vi "Periodic Tasks.vi"(8 "error in":errorcluster) -> ()   [LabVIEW 2019]
doc: "This VI runs in parallel to other tasks. It can contain as many user-defined periodic loops as you need. These can carry out PID or other sorts of timed response."
uses:
  <vilib>/Rock Robotics/WPI/Solenoid/WPI_SolenoidValue.ctl
  <vilib>/Rock Robotics/WPI/DriverStation/WPI_DriverStationRobotMode2.ctl
  Robot Global Data.vi
  <vilib>/Rock Robotics/WPI/ThirdParty/Phoenix-LabVIEW/Motor Controller/Sensor/CTRE_Phoenix_MotorControl_SetIntegratedSensorPosition_TalonFX.vi
  <vilib>/Rock Robotics/WPI/ThirdParty/Phoenix-LabVIEW/Motor Controller/Get/CTRE_Phoenix_MotorController_GetSelectedSensorData.vi
  <vilib>/Rock Robotics/WPI/Utilities/WPI_GetSetVariantRefNum.vi
  <vilib>/Rock Robotics/WPI/Solenoid/WPI_SolenoidSetEnum.vi
  <vilib>/Rock Robotics/WPI/ThirdParty/Phoenix-LabVIEW/Motor Controller/Get/CTRE_Phoenix_MotorController_GetQuadratureData.vi
  <vilib>/Rock Robotics/Network Tables/NT Read Numeric Array.vi
  <vilib>/Rock Robotics/Network Tables/NT Read String Array.vi
  <vilib>/Rock Robotics/Network Tables/NT Read Boolean Array.vi
  <vilib>/Rock Robotics/Network Tables/NT Write Numeric Array.vi
  <vilib>/Rock Robotics/Network Tables/NT Write String Array.vi
  <vilib>/Rock Robotics/Network Tables/NT Write Boolean Array.vi
  <vilib>/Rock Robotics/Network Tables/NT Read Number.vi
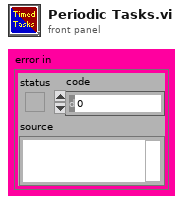
[diagram p1: front panel]
types:
  T1 = typedef "WPI_MotorControlDeviceRef.ctl" = cluster{"DeviceStatus":errorcluster, "Type":T2, "PWM":cluster{"PWM Channel":T3, "DeadBand":T4}, "CAN":cluster{"Device Number":u8, "SetOutput VI Ref":variant, "GetOutput VI Ref":variant, "Enable VI Ref":variant, "Disable VI Ref":variant, "Data":variant}, "Invert":bool, "DIO PWM":cluster{"PWM \"Enable\" Channel":T3, "DIOChannel":T5, "PWM Rate":dbl}}
  T2 = typedef "WPI_MotorControlType.ctl" = enum16{"PWM", "CAN", "DIO PWM"}
  T3 = typedef "FPGA_DIOPWMChannel.ctl" = enum8{"PWM 0", "PWM 1", "PWM 2", "PWM 3", "PWM 4", "PWM 5", "PWM 6", "PWM 7", "PWM 8", "PWM 9", "PWM MXP 0", "PWM MXP 1", "PWM MXP 2", "PWM MXP 3", "PWM MXP 4", "PWM MXP 5", "PWM MXP 6", "PWM MXP 7", "PWM MXP 8", "PWM MXP 9", "Invalid"}
  T4 = typedef "WPI_PWMDeadband.ctl" = cluster{"Name":string, "maxPositivePwm":i32, "minPositivePwm":i32, "centerPwm":i32, "maxNegativePwm":i32, "minNegativePwm":i32, "angularRange":u16}
  T5 = typedef "FPGA_DIOChannel.ctl" = enum8{"DIO 0", "DIO 1", "DIO 2", "DIO 3", "DIO 4", "DIO 5", "DIO 6", "DIO 7", "DIO 8", "DIO 9", "DIO MXP 0", "DIO MXP 1", "DIO MXP 2", "DIO MXP 3", "DIO MXP 4", "DIO MXP 5", "DIO MXP 6", "DIO MXP 7", "DIO MXP 8", "DIO MXP 9", "DIO MXP 10", "DIO MXP 11", "DIO MXP 12", "DIO MXP 13", "DIO MXP 14", "DIO MXP 15", "SPI Port CS1", "SPI Port CS2", "SPI Port CS3", "SPI Port MISO", "SPI Port MOSI", "Invalid"}
  T6 = typedef "WPI_DriverStationRobotMode2.ctl" = enum16{"Autonomous Disabled", "Autonomous Enabled", "Teleop Disabled", "Teleop Enabled", "Disconnected", "Finish", "Test Disabled", "Test Enabled", "Emergency Stopped"}
  T7 = typedef "WPI_AccelerometerDevRef.ctl" = cluster{"DevStatus":errorcluster, "Scaling":T8, "Analog Channels":T9, "I2C Bus":T11, "SPI Bus":T12, "Accel Range":T13, "ADXL Axes":T14, "Handle":i32, "Device Address":u8, "Accel Type":enum16{"Analog", "ADXL345 I2C", "ADXL345 SPI", "Internal", "ADXL362 SPI"}}
  T8 = typedef "WPI_AccelerometerScaling.ctl" = cluster{"Gain (VoltsPerG)":dbl, "Center Voltage":dbl}
  T9 = typedef "WPI_AccelerometerAnalogChannels.ctl" = cluster{"X-Axis":T10, "Y-Axis":T10, "Z-Axis":T10}
  T10 = typedef "FPGA_AIChannel.ctl" = enum8{"AI 0", "AI 1", "AI 2", "AI 3", "AI MXP 0", "AI MXP 1", "AI MXP 2", "AI MXP 3", "Invalid"}
  T11 = typedef "i2c_bus.ctl" = enum16{"I2C On-Board", "I2C MXP", "Invalid"}
  T12 = typedef "spi_bus.ctl" = enum16{"SPI On-Board, CS0", "SPI On-Board, CS1", "SPI On-Board, CS2", "SPI On-Board, CS3", "SPI MXP", "Invalid"}
  T13 = typedef "ADXL345 Range.ctl" = u8
  T14 = typedef "WPI_AccelerometerADXL345 Axes.ctl" = cluster{"X-Axis":bool, "Y-Axis":bool, "Z-Axis":bool}
  T15 = cluster{"X-Axis":dbl, "Y-Axis":dbl, "Z-Axis":dbl}
  T16 = typedef "WPI_SolenoidDevRef.ctl" = cluster{"DevStatus":errorcluster, "Pneumatics Control Module":u8, "Forward Solenoid Channel":T17, "Reverse Solenoid Channel":T17}
  T17 = typedef "WPI_SolenoidChannel.ctl" = enum8{"Solenoid 0", "Solenoid 1", "Solenoid 2", "Solenoid 3", "Solenoid 4", "Solenoid 5", "Solenoid 6", "Solenoid 7", "Invalid"}
  T18 = typedef "WPI_SolenoidValue.ctl" = enum16{"Off", "On", "Forward", "Reverse"}
  T19 = typedef "WPI_PotentiometerDevRef.ctl" = cluster{"DevStatus":errorcluster, "Analog Channel":T10, "Invert Output":bool}
  T20 = typedef "WPI_JoystickDevRef.ctl" = cluster{"Device":T21}
  T21 = typedef "WPI_JoystickDeviceEnum.ctl" = enum16{"USB 0", "USB 1", "USB 2", "USB 3", "USB 4", "USB 5"}
  T22 = typedef "Color Sensor V3 DevRef.ctl" = cluster{"I2CDevRef":T23}
  T23 = typedef "WPI_I2CDevRef.ctl" = cluster{"DevStatus":errorcluster, "Device Address":u8, "Handle":i32, "I2C Bus":T11}
  T24 = typedef "WPI_RobotDriveDevRef.ctl" = cluster{"DevStatus":errorcluster, "Motors[]":T1[], "Square Inputs":bool, "Max Output":dbl}
  T25 = cluster{"JoystickDevRef":T20, "RobotDriveDevRef":T24}
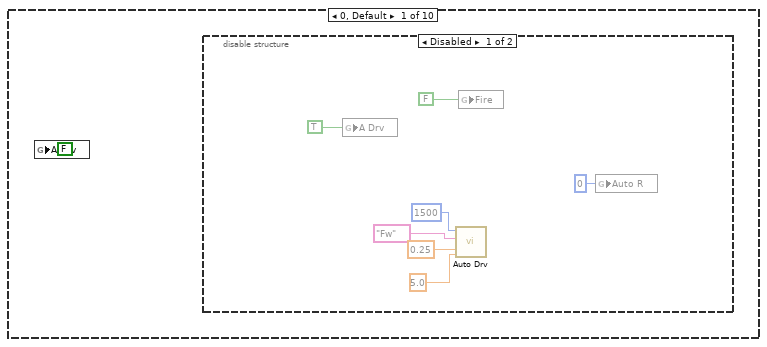
[diagram p2: hidden frame]
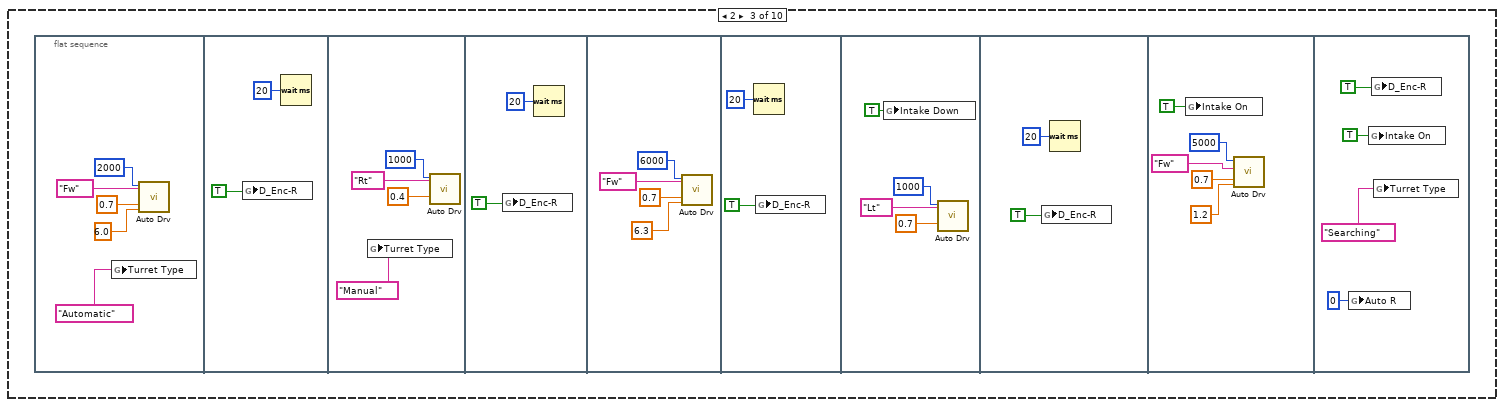
[diagram p4: hidden frame]
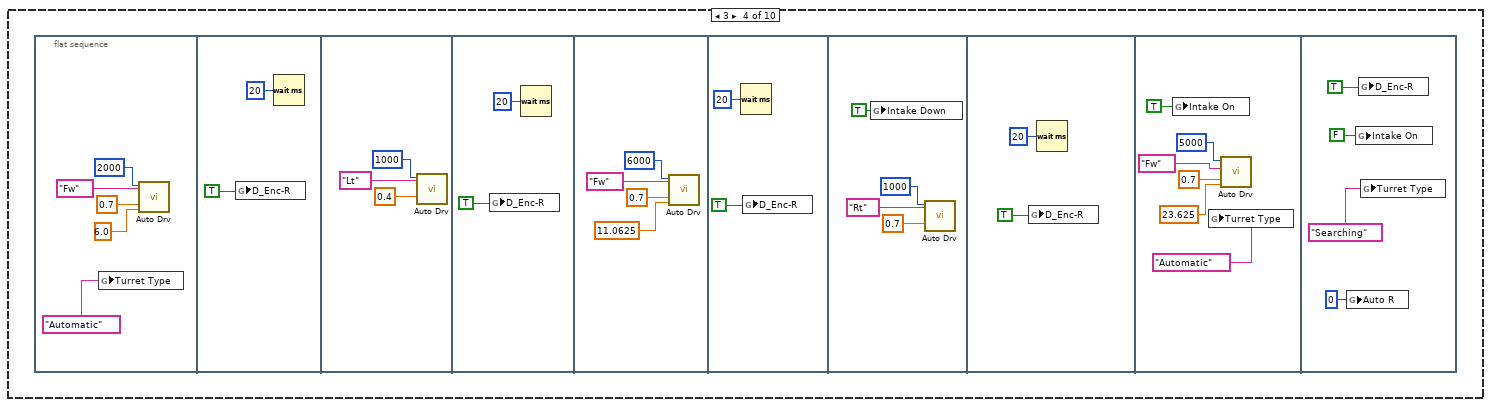
[diagram p5: hidden frame]
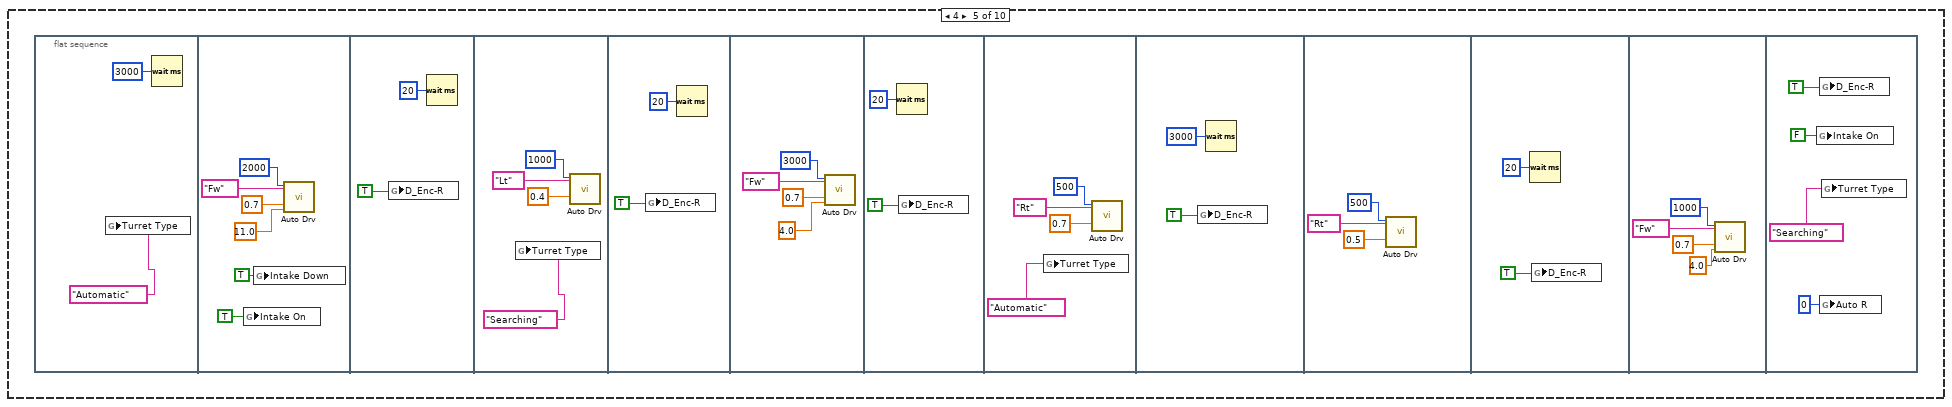
[diagram p6: hidden frame]
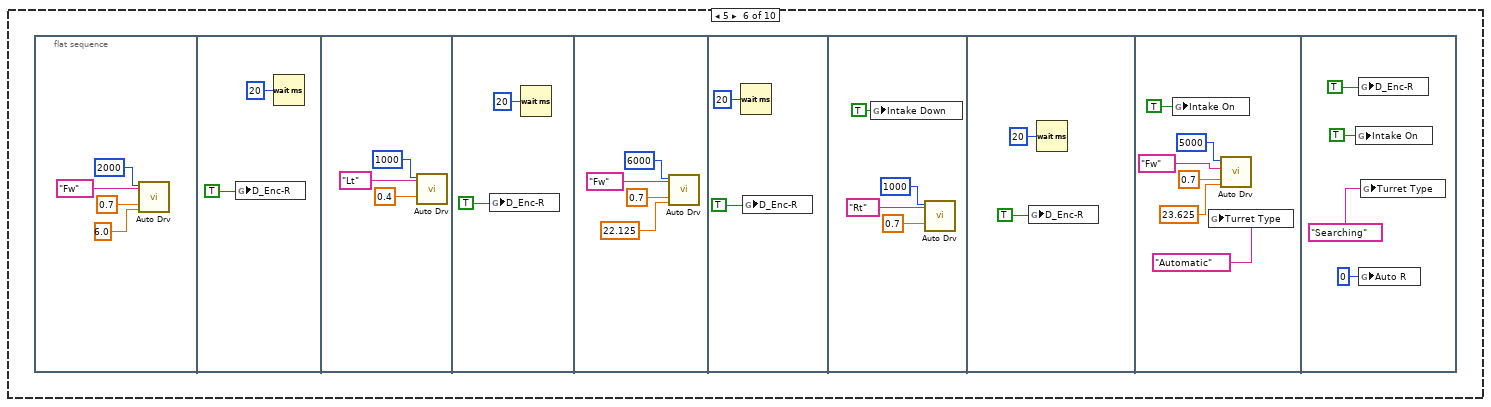
[diagram p7: hidden frame]
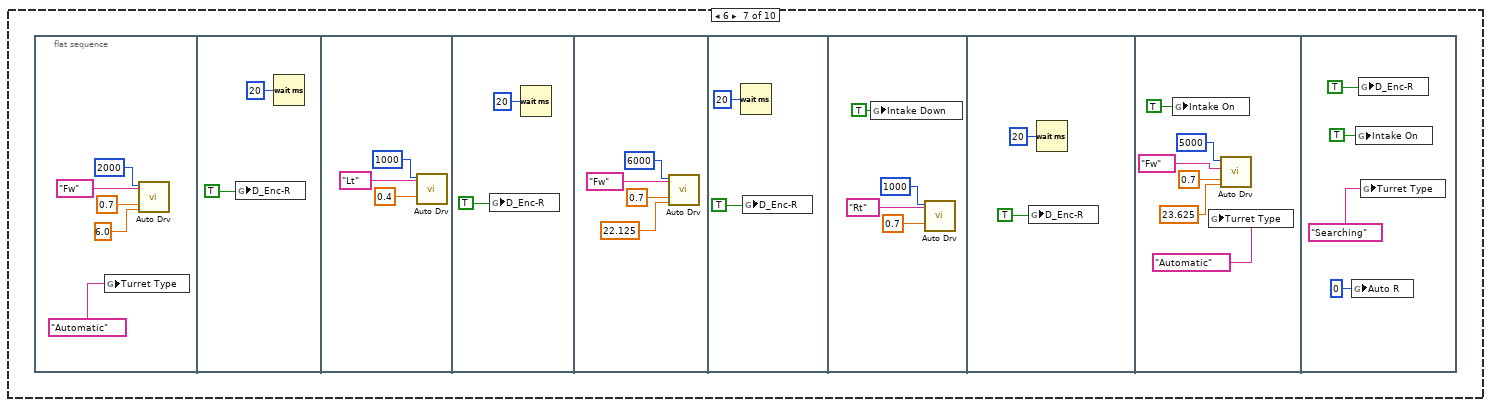
[diagram p8: hidden frame]
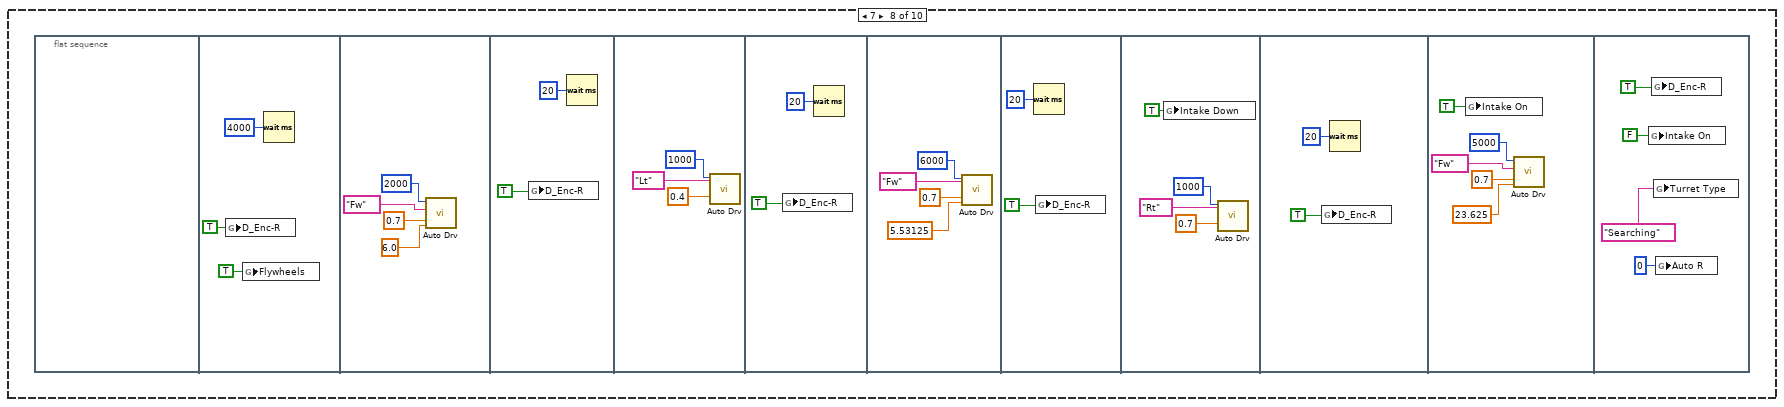
[diagram p9: hidden frame]
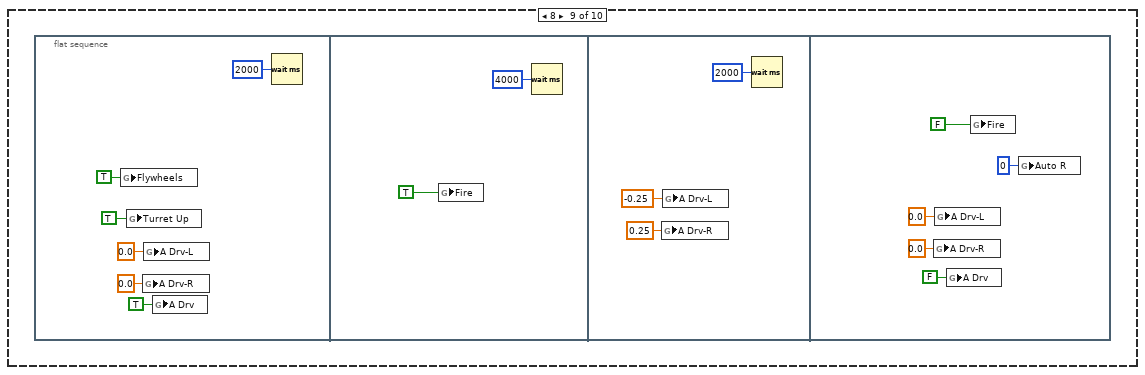
[diagram p10: hidden frame]
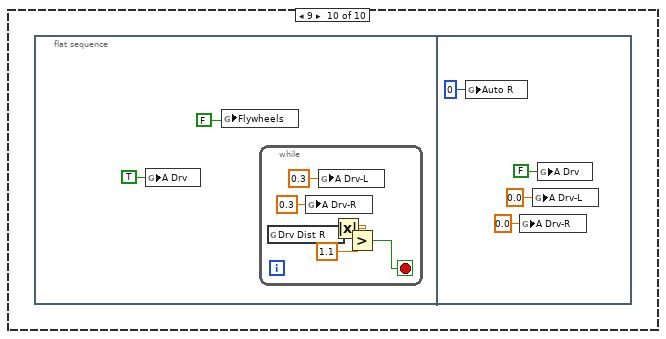
[diagram p11: hidden frame]
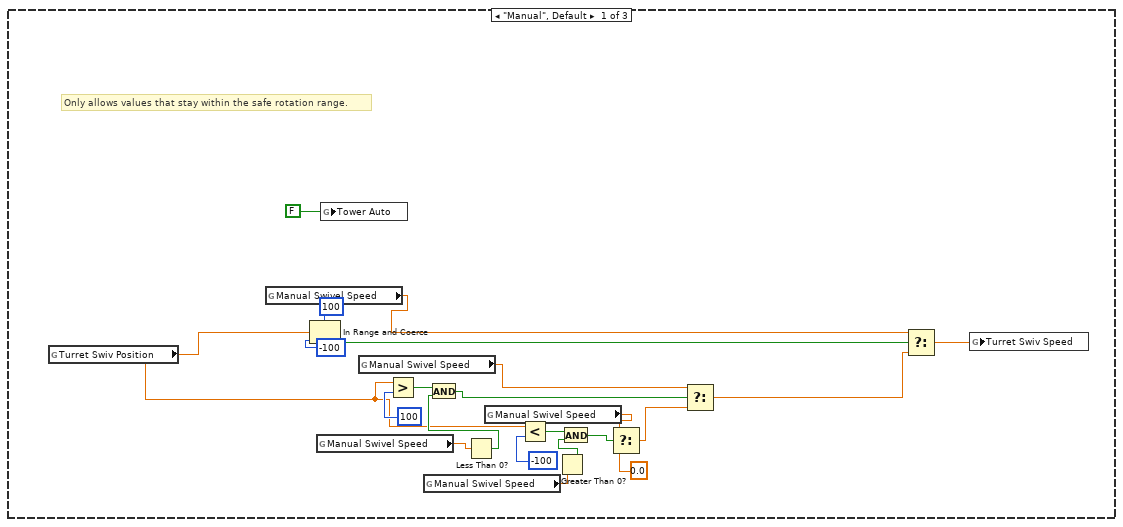
[diagram p12: hidden frame]
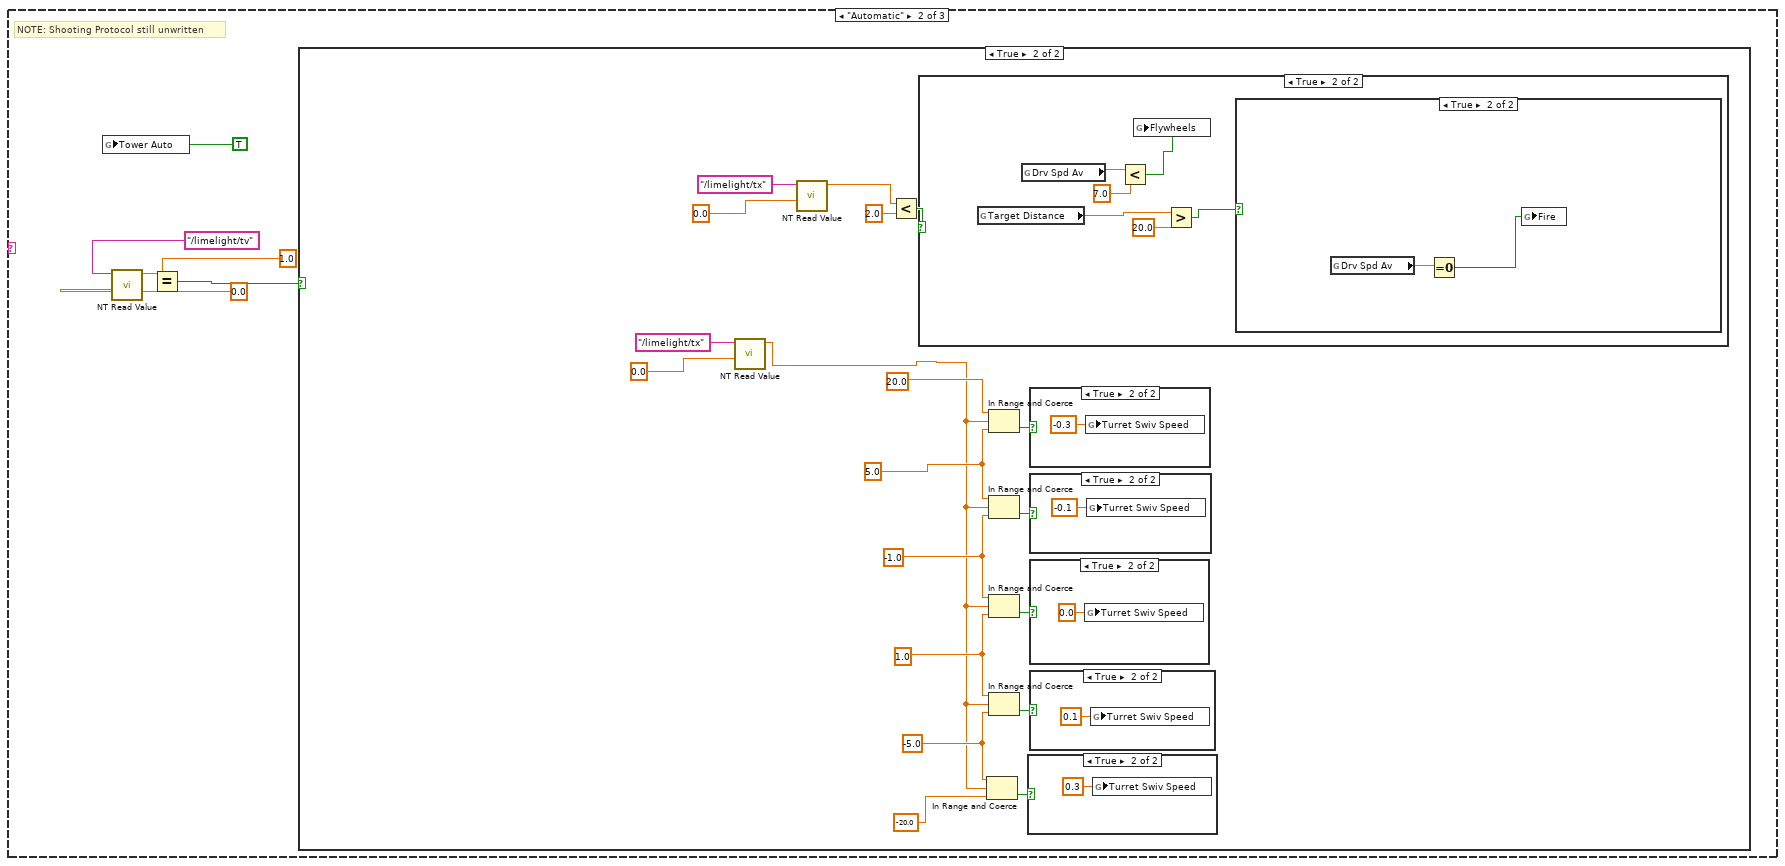
[diagram p13: hidden frame]
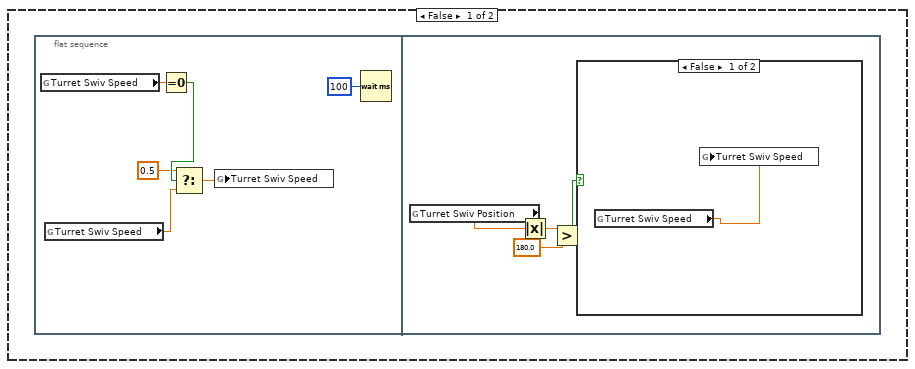
[diagram p14: hidden frame]
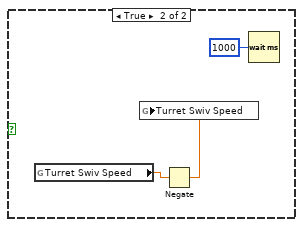
[diagram p15: hidden frame]
diagram:
  # "NOTE: All degree rotation values are not yet set. Must adjust once encoders are placeed."
  n1 = call <vilib>:"WPI_MotorControlRefNum Registry Get.vi"("refnum name"="B_Shooter 2") -> ("MotorControlDevRef"=w27:T1)  [unwired: 9 in, 1 out]
  n2 = call <vilib>:"WPI_MotorControlRefNum Registry Get.vi"("refnum name"="B_Shooter") -> ("MotorControlDevRef"=w25:T1)  [unwired: 9 in, 1 out]
  n3 = disable-structure shown="Disabled" {
    frame Disabled {
      n4 = call <vilib>:"WPI_MotorControlRefNum Registry Get.vi"("refnum name"="B_Roller") -> ("MotorControlDevRef"=w43:T1)  [unwired: 9 in, 1 out]
      n5 = while {
        tunnel: w43 -> [w47]
        tunnel: [w45] -> _
        stop <- FALSE stop-if-true
        n6 = global read "Robot Global Data.vi" "Roller Speed"() -> (w46:dbl)
        n7 = call <vilib>:"WPI_MotorControlSetOutput.vi"("Output"=w46, "MotorControlDevRef"=w47) -> ("MotorControlDevRef"=w45:T1)  [unwired: 7 in, 2 out]
        n8 = Wait (ms)(milliseconds to wait=u32 100) -> ()  [unwired: 1 out]
      }
    }
    frame Enabled {
    }
  }
  n9 = call <vilib>:"WPI_MotorControlRefNum Registry Get.vi"("refnum name"="B_Shooter") -> ("MotorControlDevRef"=w5:T1)  [unwired: 9 in, 1 out]
  n10 = call <vilib>:"WPI_MotorControlRefNum Registry Get.vi"("refnum name"="B_Shooter Swivel") -> ("MotorControlDevRef"=w20:T1)  [unwired: 9 in, 1 out]
  n11 = call <vilib>:"WPI_MotorControlRefNum Registry Get.vi"("refnum name"="B_Shooter 2") -> ("MotorControlDevRef"=w3:T1)  [unwired: 9 in, 1 out]
  n12 = disable-structure shown="Disabled" {
    frame Disabled {
      n13 = while {
        stop <- FALSE stop-if-true
        # "Tower Shift 1"
        n14 = global read "Robot Global Data.vi" "Shift Storage"() -> (w50:bool)
        n15 = case shown="True" w50 {
          frame False {
          }
          frame True {
            n16 = flat-sequence {
              frame #0 {
                n17 = global write "Robot Global Data.vi" "Tower Storage"(1.0 ("Tower Storage")) -> ()
                n18 = Wait (ms)(milliseconds to wait=u32 300) -> ()  [unwired: 1 out]
              }
              frame #1 {
                n19 = global write "Robot Global Data.vi" "Tower Storage"(0.0 ("Tower Storage")) -> ()
                n20 = global write "Robot Global Data.vi" "Shift Storage"(FALSE ("Shift Storage")) -> ()
              }
            }
          }
        }
        n21 = Wait (ms)(milliseconds to wait=u32 100) -> ()  [unwired: 1 out]
      }
    }
    frame Enabled {
    }
  }
  n22 = while {
    stop <- FALSE stop-if-true
    # "Fire Protocol"
    n23 = global read "Robot Global Data.vi" "Fire"() -> (w57:bool)
    n24 = case shown="True" w57 {
      frame False {
        n25 = global read "Robot Global Data.vi" "Tower Unjam"() -> (w61:bool)
        n26 = global read "Robot Global Data.vi" "Tower Feed On"() -> (w63:bool)
        n27 = global read "Robot Global Data.vi" "Shooter Feed On"() -> (w64:bool)
        n28 = global read "Robot Global Data.vi" "Shooter Feed"() -> (w66:dbl)
        n29 = global read "Robot Global Data.vi" "Tower Storage"() -> (w69:dbl)
        n30 = Or(x=w63, y=w61) -> (x .or. y?=w62:bool)
        n31 = Or(x=w61, y=w64) -> (x .or. y?=w60:bool)
        n32 = Select(t=w66, s=w60, f=0.0) -> (s? t:f=w67:dbl)
        n33 = Select(t=w69, s=w62, f=0.0) -> (s? t:f=w68:dbl)
        n34 = global write "Robot Global Data.vi" "Shooter Feed"(w67) -> ()
        n35 = global write "Robot Global Data.vi" "Tower Storage"(w68) -> ()
      }
      frame True {
        n36 = global write "Robot Global Data.vi" "Shooter Feed"(1.0 ("Tower Storage")) -> ()
        n37 = global write "Robot Global Data.vi" "Tower Storage"(1.0 ("Tower Storage")) -> ()
        n38 = global write "Robot Global Data.vi" "Tower Feed On"(FALSE ("Tower Feed On")) -> ()
      }
    }
    n39 = Wait (ms)(milliseconds to wait=u32 100) -> ()  [unwired: 1 out]
  }
  n40 = while {
    stop <- FALSE stop-if-true
    # "Autonomous Code"
    n41 = call <vilib>:"WPI_DriverStationGetModeAndStatus.vi"() -> ("Robot Mode"=w79:T6)  [unwired: 10 in, 1 out]
    n42 = global read "Robot Global Data.vi" "Auto R"() -> (w74:i8)
    n43 = Equal?(x=w79, y=WPI_DriverStationRobotMode2."Teleop Enabled") -> (x = y?=w77:bool)
    n44 = global read "Robot Global Data.vi" "Auto R"() -> (w80:i8)
    n45 = Select(t=0.0, s=w77, f=w74) -> (s? t:f=w75:dbl)
    n46 = global write "Robot Global Data.vi" "Auto R"(w75) -> ()
    n47 = case shown="1" w80 {
      frame 0, Default {
        n48 = global write "Robot Global Data.vi" "A Drv"(FALSE ("Flywheels")) -> ()
        n49 = disable-structure shown="Disabled" {
          frame Disabled {
            n50 = global write "Robot Global Data.vi" "A Drv"(TRUE ("Flywheels")) -> ()
            n51 = call "Auto Drv.vi"("Time Out ms"=1500, "Direction"="Fw", "Power"=0.25 ("Distance Ft"), "Distance Ft"=5.0) -> ()  [unwired: 6 in]
            n52 = global write "Robot Global Data.vi" "Fire"(FALSE ("Flywheels")) -> ()
            n53 = global write "Robot Global Data.vi" "Auto R"(i8 0 ("Auto R")) -> ()
          }
          frame Enabled {
          }
        }
      }
      frame 1 {
        n54 = flat-sequence {
          frame #0 {
            n55 = global write "Robot Global Data.vi" "Flywheels"(TRUE ("Flywheels")) -> ()
            n56 = global write "Robot Global Data.vi" "Turret Up"(TRUE ("Flywheels")) -> ()
            n57 = global write "Robot Global Data.vi" "A Drv-R"(0.0 ("A Drv-L")) -> ()
            n58 = global write "Robot Global Data.vi" "A Drv-L"(0.0 ("A Drv-L")) -> ()
            n59 = global write "Robot Global Data.vi" "A Drv"(TRUE ("A Drv")) -> ()
            n60 = Wait (ms)(milliseconds to wait=u32 500) -> ()  [unwired: 1 out]
          }
          frame #1 {
            n61 = global write "Robot Global Data.vi" "Fire"(TRUE ("Flywheels")) -> ()
            n62 = Wait (ms)(milliseconds to wait=u32 4000) -> ()  [unwired: 1 out]
          }
          frame #2 {
            n63 = global write "Robot Global Data.vi" "Flywheels"(FALSE ("Flywheels")) -> ()
            n64 = global write "Robot Global Data.vi" "Fire"(FALSE ("Flywheels")) -> ()
            n65 = global write "Robot Global Data.vi" "A Drv-R"(0.25 ("A Drv-L")) -> ()
            n66 = global write "Robot Global Data.vi" "A Drv-L"(-0.25 ("A Drv-L")) -> ()
            n67 = Wait (ms)(milliseconds to wait=u32 2000) -> ()  [unwired: 1 out]
          }
          frame #3 {
            n68 = global write "Robot Global Data.vi" "D_Enc-R"(TRUE ("D_Enc-R")) -> ()
            n69 = global write "Robot Global Data.vi" "A Drv-R"(0.0 ("A Drv-L")) -> ()
            n70 = global write "Robot Global Data.vi" "A Drv-L"(0.0 ("A Drv-L")) -> ()
            n71 = Wait (ms)(milliseconds to wait=u32 200) -> ()  [unwired: 1 out]
          }
          frame #4 {
            n72 = while {
              stop <- w110 stop-if-true
              n73 = global read "Robot Global Data.vi" "Drv Dist R"() -> (w108:dbl)
              n74 = global write "Robot Global Data.vi" "A Drv-R"(0.3 ("A Drv-L")) -> ()
              n75 = global write "Robot Global Data.vi" "A Drv-L"(0.3 ("A Drv-L")) -> ()
              n76 = Absolute Value(x=w108) -> (abs(x)=w109:dbl)
              n77 = Greater?(x=w109, y=1.1) -> (0:w110:bool)
            }
          }
          frame #5 {
            n78 = global write "Robot Global Data.vi" "D_Enc-R"(TRUE ("D_Enc-R")) -> ()
            n79 = global write "Robot Global Data.vi" "A Drv-R"(0.0 ("A Drv-L")) -> ()
            n80 = global write "Robot Global Data.vi" "A Drv-L"(0.0 ("A Drv-L")) -> ()
            n81 = Wait (ms)(milliseconds to wait=u32 200) -> ()  [unwired: 1 out]
          }
          frame #6 {
            n82 = while {
              stop <- w121 stop-if-true
              n83 = global read "Robot Global Data.vi" "Drv Dist Av"() -> (w118:dbl)
              n84 = global write "Robot Global Data.vi" "A Drv-R"(-0.3 ("A Drv-L")) -> ()
              n85 = global write "Robot Global Data.vi" "A Drv-L"(0.3 ("A Drv-L")) -> ()
              n86 = Absolute Value(x=w118) -> (abs(x)=w119:dbl)
              n87 = Greater?(x=w119, y=6.25) -> (0:w121:bool)
            }
          }
          frame #7 {
            n88 = global write "Robot Global Data.vi" "D_Enc-R"(TRUE ("D_Enc-R")) -> ()
            n89 = global write "Robot Global Data.vi" "A Drv-R"(0.0 ("A Drv-L")) -> ()
            n90 = global write "Robot Global Data.vi" "A Drv-L"(0.0 ("A Drv-L")) -> ()
            n91 = Wait (ms)(milliseconds to wait=u32 200) -> ()  [unwired: 1 out]
          }
          frame #8 {
            n92 = while {
              stop <- w131 stop-if-true
              n93 = global read "Robot Global Data.vi" "Drv Dist R"() -> (w129:dbl)
              n94 = global write "Robot Global Data.vi" "A Drv-R"(0.3 ("A Drv-L")) -> ()
              n95 = global write "Robot Global Data.vi" "A Drv-L"(0.3 ("A Drv-L")) -> ()
              n96 = Absolute Value(x=w129) -> (abs(x)=w130:dbl)
              n97 = Greater?(x=w130, y=1.1) -> (0:w131:bool)
            }
            n98 = global write "Robot Global Data.vi" "Intake Down"(TRUE ("Flywheels")) -> ()
          }
          frame #9 {
            n99 = global write "Robot Global Data.vi" "D_Enc-R"(TRUE ("D_Enc-R")) -> ()
            n100 = global write "Robot Global Data.vi" "A Drv-R"(0.0 ("A Drv-L")) -> ()
            n101 = global write "Robot Global Data.vi" "A Drv-L"(0.0 ("A Drv-L")) -> ()
            n102 = Wait (ms)(milliseconds to wait=u32 200) -> ()  [unwired: 1 out]
          }
          frame #10 {
            n103 = while {
              stop <- w142 stop-if-true
              n104 = global read "Robot Global Data.vi" "Drv Dist Av"() -> (w140:dbl)
              n105 = global write "Robot Global Data.vi" "A Drv-R"(-0.3 ("A Drv-L")) -> ()
              n106 = global write "Robot Global Data.vi" "A Drv-L"(0.3 ("A Drv-L")) -> ()
              n107 = Absolute Value(x=w140) -> (abs(x)=w141:dbl)
              n108 = Greater?(x=w141, y=23.625) -> (0:w142:bool)
            }
            n109 = global write "Robot Global Data.vi" "Intake On"(TRUE ("Flywheels")) -> ()
          }
          frame #11 {
            n110 = global write "Robot Global Data.vi" "A Drv-R"(0.0 ("A Drv-L")) -> ()
            n111 = global write "Robot Global Data.vi" "D_Enc-R"(TRUE ("D_Enc-R")) -> ()
            n112 = global write "Robot Global Data.vi" "A Drv-L"(0.0 ("A Drv-L")) -> ()
            n113 = Wait (ms)(milliseconds to wait=u32 200) -> ()  [unwired: 1 out]
          }
          frame #12 {
            n114 = Wait (ms)(milliseconds to wait=u32 500) -> ()  [unwired: 1 out]
            n115 = global write "Robot Global Data.vi" "A Drv-R"(0.3 ("A Drv-L")) -> ()
            n116 = global write "Robot Global Data.vi" "A Drv-L"(0.3 ("A Drv-L")) -> ()
          }
          frame #13 {
            n117 = while {
              stop <- w161 stop-if-true
              n118 = global read "Robot Global Data.vi" "Turret Swiv Position"() -> (w163:dbl)
              n119 = call-poly <vilib>:"NT Read Value.vi"("Default Value"=0.0, "Name"="/limelight/tv") -> ("Numeric"=w157:dbl)  [unwired: 8 in, 1 out]
              n120 = call-poly <vilib>:"NT Read Value.vi"("Default Value"=0.0, "Name"="/limelight/tx") -> ("Numeric"=w168:dbl)  [unwired: 8 in, 1 out]
              n121 = Equal?(x=w157, y=1.0) -> (x = y?=w155:bool)
              n122 = global write "Robot Global Data.vi" "Manual Swivel Speed"(0.6 ("Manual Swivel Speed")) -> ()
              n123 = Less?(x=w168, y=2.0) -> (x < y?=w160:bool)
              n124 = Greater?(x=w163, y=130.0) -> (0:w164:bool)
              n125 = global write "Robot Global Data.vi" "A Drv-R"(0.0 ("A Drv-L")) -> ()
              n126 = global write "Robot Global Data.vi" "A Drv-L"(0.0 ("A Drv-L")) -> ()
              n127 = And(x=w155, y=w160) -> (x .and. y?=w154:bool)
              n128 = Or(x=w154, y=w164) -> (x .or. y?=w161:bool)
            }
            n129 = global write "Robot Global Data.vi" "D_Enc-R"(TRUE ("D_Enc-R")) -> ()
          }
          frame #14 {
            n130 = global write "Robot Global Data.vi" "Manual Swivel Speed"(0.0 ("Manual Swivel Speed")) -> ()
            n131 = global write "Robot Global Data.vi" "Auto R"(i8 0 ("Auto R")) -> ()
            n132 = global write "Robot Global Data.vi" "Flywheels"(TRUE ("Flywheels")) -> ()
            n133 = global write "Robot Global Data.vi" "Intake On"(FALSE ("Flywheels")) -> ()
            n134 = global write "Robot Global Data.vi" "A Drv"(FALSE ("A Drv")) -> ()
          }
        }
      }
      frame 2 {
        n135 = flat-sequence {
          frame #0 {
            n136 = global write "Robot Global Data.vi" "Turret Type"("Automatic" ("Turret Mode")) -> ()
            n137 = call "Auto Drv.vi"("Time Out ms"=2000, "Direction"="Fw", "Power"=0.7 ("Distance Ft"), "Distance Ft"=6.0) -> ()  [unwired: 6 in]
          }
          frame #1 {
            n138 = global write "Robot Global Data.vi" "D_Enc-R"(TRUE ("D_Enc-R")) -> ()
            n139 = Wait (ms)(milliseconds to wait=u32 20) -> ()  [unwired: 1 out]
          }
          frame #2 {
            n140 = global write "Robot Global Data.vi" "Turret Type"("Manual" ("Turret Mode")) -> ()
            n141 = call "Auto Drv.vi"("Time Out ms"=1000, "Direction"="Rt", "Power"=0.4 ("Distance Ft")) -> ()  [unwired: 7 in]
          }
          frame #3 {
            n142 = global write "Robot Global Data.vi" "D_Enc-R"(TRUE ("D_Enc-R")) -> ()
            n143 = Wait (ms)(milliseconds to wait=u32 20) -> ()  [unwired: 1 out]
          }
          frame #4 {
            n144 = call "Auto Drv.vi"("Time Out ms"=6000, "Direction"="Fw", "Power"=0.7 ("Distance Ft"), "Distance Ft"=6.3) -> ()  [unwired: 6 in]
          }
          frame #5 {
            n145 = Wait (ms)(milliseconds to wait=u32 20) -> ()  [unwired: 1 out]
            n146 = global write "Robot Global Data.vi" "D_Enc-R"(TRUE ("D_Enc-R")) -> ()
          }
          frame #6 {
            n147 = global write "Robot Global Data.vi" "Intake Down"(TRUE ("Intake Down")) -> ()
            n148 = call "Auto Drv.vi"("Time Out ms"=1000, "Direction"="Lt", "Power"=0.7 ("Distance Ft")) -> ()  [unwired: 7 in]
          }
          frame #7 {
            n149 = global write "Robot Global Data.vi" "D_Enc-R"(TRUE ("D_Enc-R")) -> ()
            n150 = Wait (ms)(milliseconds to wait=u32 20) -> ()  [unwired: 1 out]
          }
          frame #8 {
            n151 = global write "Robot Global Data.vi" "Intake On"(TRUE ("Intake Down")) -> ()
            n152 = call "Auto Drv.vi"("Time Out ms"=5000, "Direction"="Fw", "Power"=0.7 ("Distance Ft"), "Distance Ft"=1.2) -> ()  [unwired: 6 in]
          }
          frame #9 {
            n153 = global write "Robot Global Data.vi" "Auto R"(i8 0 ("Auto R")) -> ()
            n154 = global write "Robot Global Data.vi" "Intake On"(TRUE ("Intake Down")) -> ()
            n155 = global write "Robot Global Data.vi" "D_Enc-R"(TRUE ("D_Enc-R")) -> ()
            n156 = global write "Robot Global Data.vi" "Turret Type"("Searching" ("Turret Mode")) -> ()
          }
        }
      }
      frame 3 {
        n157 = flat-sequence {
          frame #0 {
            n158 = global write "Robot Global Data.vi" "Turret Type"("Automatic" ("Turret Mode")) -> ()
            n159 = call "Auto Drv.vi"("Time Out ms"=2000, "Direction"="Fw", "Power"=0.7 ("Distance Ft"), "Distance Ft"=6.0) -> ()  [unwired: 6 in]
          }
          frame #1 {
            n160 = global write "Robot Global Data.vi" "D_Enc-R"(TRUE ("D_Enc-R")) -> ()
            n161 = Wait (ms)(milliseconds to wait=u32 20) -> ()  [unwired: 1 out]
          }
          frame #2 {
            n162 = call "Auto Drv.vi"("Time Out ms"=1000, "Direction"="Lt", "Power"=0.4 ("Distance Ft")) -> ()  [unwired: 7 in]
          }
          frame #3 {
            n163 = global write "Robot Global Data.vi" "D_Enc-R"(TRUE ("D_Enc-R")) -> ()
            n164 = Wait (ms)(milliseconds to wait=u32 20) -> ()  [unwired: 1 out]
          }
          frame #4 {
            n165 = call "Auto Drv.vi"("Time Out ms"=6000, "Direction"="Fw", "Power"=0.7 ("Distance Ft"), "Distance Ft"=11.0625) -> ()  [unwired: 6 in]
          }
          frame #5 {
            n166 = Wait (ms)(milliseconds to wait=u32 20) -> ()  [unwired: 1 out]
            n167 = global write "Robot Global Data.vi" "D_Enc-R"(TRUE ("D_Enc-R")) -> ()
          }
          frame #6 {
            n168 = global write "Robot Global Data.vi" "Intake Down"(TRUE ("Intake Down")) -> ()
            n169 = call "Auto Drv.vi"("Time Out ms"=1000, "Direction"="Rt", "Power"=0.7 ("Distance Ft")) -> ()  [unwired: 7 in]
          }
          frame #7 {
            n170 = global write "Robot Global Data.vi" "D_Enc-R"(TRUE ("D_Enc-R")) -> ()
            n171 = Wait (ms)(milliseconds to wait=u32 20) -> ()  [unwired: 1 out]
          }
          frame #8 {
            n172 = global write "Robot Global Data.vi" "Intake On"(TRUE ("Intake Down")) -> ()
            n173 = global write "Robot Global Data.vi" "Turret Type"("Automatic" ("Turret Mode")) -> ()
            n174 = call "Auto Drv.vi"("Time Out ms"=5000, "Direction"="Fw", "Power"=0.7 ("Distance Ft"), "Distance Ft"=23.625) -> ()  [unwired: 6 in]
          }
          frame #9 {
            n175 = global write "Robot Global Data.vi" "Auto R"(i8 0 ("Auto R")) -> ()
            n176 = global write "Robot Global Data.vi" "Intake On"(FALSE ("Intake Down")) -> ()
            n177 = global write "Robot Global Data.vi" "D_Enc-R"(TRUE ("D_Enc-R")) -> ()
            n178 = global write "Robot Global Data.vi" "Turret Type"("Searching" ("Turret Mode")) -> ()
          }
        }
      }
      frame 4 {
        n179 = flat-sequence {
          frame #0 {
            n180 = global write "Robot Global Data.vi" "Turret Type"("Automatic" ("Turret Mode")) -> ()
            n181 = Wait (ms)(milliseconds to wait=u32 3000) -> ()  [unwired: 1 out]
          }
          frame #1 {
            n182 = global write "Robot Global Data.vi" "Intake On"(TRUE ("Intake Down")) -> ()
            n183 = global write "Robot Global Data.vi" "Intake Down"(TRUE ("Intake Down")) -> ()
            n184 = call "Auto Drv.vi"("Time Out ms"=2000, "Direction"="Fw", "Power"=0.7 ("Distance Ft"), "Distance Ft"=11.0) -> ()  [unwired: 6 in]
          }
          frame #2 {
            n185 = global write "Robot Global Data.vi" "D_Enc-R"(TRUE ("D_Enc-R")) -> ()
            n186 = Wait (ms)(milliseconds to wait=u32 20) -> ()  [unwired: 1 out]
          }
          frame #3 {
            n187 = global write "Robot Global Data.vi" "Turret Type"("Searching" ("Turret Mode")) -> ()
            n188 = call "Auto Drv.vi"("Time Out ms"=1000, "Direction"="Lt", "Power"=0.4 ("Distance Ft")) -> ()  [unwired: 7 in]
          }
          frame #4 {
            n189 = global write "Robot Global Data.vi" "D_Enc-R"(TRUE ("D_Enc-R")) -> ()
            n190 = Wait (ms)(milliseconds to wait=u32 20) -> ()  [unwired: 1 out]
          }
          frame #5 {
            n191 = call "Auto Drv.vi"("Time Out ms"=3000, "Direction"="Fw", "Power"=0.7 ("Distance Ft"), "Distance Ft"=4.0) -> ()  [unwired: 6 in]
          }
          frame #6 {
            n192 = Wait (ms)(milliseconds to wait=u32 20) -> ()  [unwired: 1 out]
            n193 = global write "Robot Global Data.vi" "D_Enc-R"(TRUE ("D_Enc-R")) -> ()
          }
          frame #7 {
            n194 = global write "Robot Global Data.vi" "Turret Type"("Automatic" ("Turret Mode")) -> ()
            n195 = call "Auto Drv.vi"("Time Out ms"=500, "Direction"="Rt", "Power"=0.7 ("Distance Ft")) -> ()  [unwired: 7 in]
          }
          frame #8 {
            n196 = global write "Robot Global Data.vi" "D_Enc-R"(TRUE ("D_Enc-R")) -> ()
            n197 = Wait (ms)(milliseconds to wait=u32 3000) -> ()  [unwired: 1 out]
          }
          frame #9 {
            n198 = call "Auto Drv.vi"("Time Out ms"=500, "Direction"="Rt", "Power"=0.5 ("Distance Ft")) -> ()  [unwired: 7 in]
          }
          frame #10 {
            n199 = Wait (ms)(milliseconds to wait=u32 20) -> ()  [unwired: 1 out]
            n200 = global write "Robot Global Data.vi" "D_Enc-R"(TRUE ("D_Enc-R")) -> ()
          }
          frame #11 {
            n201 = call "Auto Drv.vi"("Time Out ms"=1000, "Direction"="Fw", "Power"=0.7 ("Distance Ft"), "Distance Ft"=4.0) -> ()  [unwired: 6 in]
          }
          frame #12 {
            n202 = global write "Robot Global Data.vi" "Intake On"(FALSE ("Intake Down")) -> ()
            n203 = global write "Robot Global Data.vi" "D_Enc-R"(TRUE ("D_Enc-R")) -> ()
            n204 = global write "Robot Global Data.vi" "Auto R"(i8 0 ("Auto R")) -> ()
            n205 = global write "Robot Global Data.vi" "Turret Type"("Searching" ("Turret Mode")) -> ()
          }
        }
      }
      frame 5 {
        n206 = flat-sequence {
          frame #0 {
            n207 = call "Auto Drv.vi"("Time Out ms"=2000, "Direction"="Fw", "Power"=0.7 ("Distance Ft"), "Distance Ft"=6.0) -> ()  [unwired: 6 in]
          }
          frame #1 {
            n208 = global write "Robot Global Data.vi" "D_Enc-R"(TRUE ("D_Enc-R")) -> ()
            n209 = Wait (ms)(milliseconds to wait=u32 20) -> ()  [unwired: 1 out]
          }
          frame #2 {
            n210 = call "Auto Drv.vi"("Time Out ms"=1000, "Direction"="Lt", "Power"=0.4 ("Distance Ft")) -> ()  [unwired: 7 in]
          }
          frame #3 {
            n211 = global write "Robot Global Data.vi" "D_Enc-R"(TRUE ("D_Enc-R")) -> ()
            n212 = Wait (ms)(milliseconds to wait=u32 20) -> ()  [unwired: 1 out]
          }
          frame #4 {
            n213 = call "Auto Drv.vi"("Time Out ms"=6000, "Direction"="Fw", "Power"=0.7 ("Distance Ft"), "Distance Ft"=22.125) -> ()  [unwired: 6 in]
          }
          frame #5 {
            n214 = Wait (ms)(milliseconds to wait=u32 20) -> ()  [unwired: 1 out]
            n215 = global write "Robot Global Data.vi" "D_Enc-R"(TRUE ("D_Enc-R")) -> ()
          }
          frame #6 {
            n216 = global write "Robot Global Data.vi" "Intake Down"(TRUE ("Intake Down")) -> ()
            n217 = call "Auto Drv.vi"("Time Out ms"=1000, "Direction"="Rt", "Power"=0.7 ("Distance Ft")) -> ()  [unwired: 7 in]
          }
          frame #7 {
            n218 = global write "Robot Global Data.vi" "D_Enc-R"(TRUE ("D_Enc-R")) -> ()
            n219 = Wait (ms)(milliseconds to wait=u32 20) -> ()  [unwired: 1 out]
          }
          frame #8 {
            n220 = global write "Robot Global Data.vi" "Intake On"(TRUE ("Intake Down")) -> ()
            n221 = global write "Robot Global Data.vi" "Turret Type"("Automatic" ("Turret Mode")) -> ()
            n222 = call "Auto Drv.vi"("Time Out ms"=5000, "Direction"="Fw", "Power"=0.7 ("Distance Ft"), "Distance Ft"=23.625) -> ()  [unwired: 6 in]
          }
          frame #9 {
            n223 = global write "Robot Global Data.vi" "Intake On"(TRUE ("Intake Down")) -> ()
            n224 = global write "Robot Global Data.vi" "D_Enc-R"(TRUE ("D_Enc-R")) -> ()
            n225 = global write "Robot Global Data.vi" "Auto R"(i8 0 ("Auto R")) -> ()
            n226 = global write "Robot Global Data.vi" "Turret Type"("Searching" ("Turret Mode")) -> ()
          }
        }
      }
      frame 6 {
        n227 = flat-sequence {
          frame #0 {
            n228 = global write "Robot Global Data.vi" "Turret Type"("Automatic" ("Turret Mode")) -> ()
            n229 = call "Auto Drv.vi"("Time Out ms"=2000, "Direction"="Fw", "Power"=0.7 ("Distance Ft"), "Distance Ft"=6.0) -> ()  [unwired: 6 in]
          }
          frame #1 {
            n230 = global write "Robot Global Data.vi" "D_Enc-R"(TRUE ("D_Enc-R")) -> ()
            n231 = Wait (ms)(milliseconds to wait=u32 20) -> ()  [unwired: 1 out]
          }
          frame #2 {
            n232 = call "Auto Drv.vi"("Time Out ms"=1000, "Direction"="Lt", "Power"=0.4 ("Distance Ft")) -> ()  [unwired: 7 in]
          }
          frame #3 {
            n233 = global write "Robot Global Data.vi" "D_Enc-R"(TRUE ("D_Enc-R")) -> ()
            n234 = Wait (ms)(milliseconds to wait=u32 20) -> ()  [unwired: 1 out]
          }
          frame #4 {
            n235 = call "Auto Drv.vi"("Time Out ms"=6000, "Direction"="Fw", "Power"=0.7 ("Distance Ft"), "Distance Ft"=22.125) -> ()  [unwired: 6 in]
          }
          frame #5 {
            n236 = Wait (ms)(milliseconds to wait=u32 20) -> ()  [unwired: 1 out]
            n237 = global write "Robot Global Data.vi" "D_Enc-R"(TRUE ("D_Enc-R")) -> ()
          }
          frame #6 {
            n238 = global write "Robot Global Data.vi" "Intake Down"(TRUE ("Intake Down")) -> ()
            n239 = call "Auto Drv.vi"("Time Out ms"=1000, "Direction"="Rt", "Power"=0.7 ("Distance Ft")) -> ()  [unwired: 7 in]
          }
          frame #7 {
            n240 = global write "Robot Global Data.vi" "D_Enc-R"(TRUE ("D_Enc-R")) -> ()
            n241 = Wait (ms)(milliseconds to wait=u32 20) -> ()  [unwired: 1 out]
          }
          frame #8 {
            n242 = global write "Robot Global Data.vi" "Intake On"(TRUE ("Intake Down")) -> ()
            n243 = global write "Robot Global Data.vi" "Turret Type"("Automatic" ("Turret Mode")) -> ()
            n244 = call "Auto Drv.vi"("Time Out ms"=5000, "Direction"="Fw", "Power"=0.7 ("Distance Ft"), "Distance Ft"=23.625) -> ()  [unwired: 6 in]
          }
          frame #9 {
            n245 = global write "Robot Global Data.vi" "Auto R"(i8 0 ("Auto R")) -> ()
            n246 = global write "Robot Global Data.vi" "Intake On"(TRUE ("Intake Down")) -> ()
            n247 = global write "Robot Global Data.vi" "D_Enc-R"(TRUE ("D_Enc-R")) -> ()
            n248 = global write "Robot Global Data.vi" "Turret Type"("Searching" ("Turret Mode")) -> ()
          }
        }
      }
      frame 7 {
        n249 = flat-sequence {
          frame #0 {
          }
          frame #1 {
            n250 = global write "Robot Global Data.vi" "D_Enc-R"(TRUE ("D_Enc-R")) -> ()
            n251 = global write "Robot Global Data.vi" "Flywheels"(TRUE ("Flywheels")) -> ()
            n252 = Wait (ms)(milliseconds to wait=u32 4000) -> ()  [unwired: 1 out]
          }
          frame #2 {
            n253 = call "Auto Drv.vi"("Time Out ms"=2000, "Direction"="Fw", "Power"=0.7 ("Distance Ft"), "Distance Ft"=6.0) -> ()  [unwired: 6 in]
          }
          frame #3 {
            n254 = global write "Robot Global Data.vi" "D_Enc-R"(TRUE ("D_Enc-R")) -> ()
            n255 = Wait (ms)(milliseconds to wait=u32 20) -> ()  [unwired: 1 out]
          }
          frame #4 {
            n256 = call "Auto Drv.vi"("Time Out ms"=1000, "Direction"="Lt", "Power"=0.4 ("Distance Ft")) -> ()  [unwired: 7 in]
          }
          frame #5 {
            n257 = global write "Robot Global Data.vi" "D_Enc-R"(TRUE ("D_Enc-R")) -> ()
            n258 = Wait (ms)(milliseconds to wait=u32 20) -> ()  [unwired: 1 out]
          }
          frame #6 {
            n259 = call "Auto Drv.vi"("Time Out ms"=6000, "Direction"="Fw", "Power"=0.7 ("Distance Ft"), "Distance Ft"=5.53125) -> ()  [unwired: 6 in]
          }
          frame #7 {
            n260 = Wait (ms)(milliseconds to wait=u32 20) -> ()  [unwired: 1 out]
            n261 = global write "Robot Global Data.vi" "D_Enc-R"(TRUE ("D_Enc-R")) -> ()
          }
          frame #8 {
            n262 = global write "Robot Global Data.vi" "Intake Down"(TRUE ("Intake Down")) -> ()
            n263 = call "Auto Drv.vi"("Time Out ms"=1000, "Direction"="Rt", "Power"=0.7 ("Distance Ft")) -> ()  [unwired: 7 in]
          }
          frame #9 {
            n264 = global write "Robot Global Data.vi" "D_Enc-R"(TRUE ("D_Enc-R")) -> ()
            n265 = Wait (ms)(milliseconds to wait=u32 20) -> ()  [unwired: 1 out]
          }
          frame #10 {
            n266 = global write "Robot Global Data.vi" "Intake On"(TRUE ("Intake Down")) -> ()
            n267 = call "Auto Drv.vi"("Time Out ms"=5000, "Direction"="Fw", "Power"=0.7 ("Distance Ft"), "Distance Ft"=23.625) -> ()  [unwired: 6 in]
          }
          frame #11 {
            n268 = global write "Robot Global Data.vi" "Intake On"(FALSE ("Intake Down")) -> ()
            n269 = global write "Robot Global Data.vi" "D_Enc-R"(TRUE ("D_Enc-R")) -> ()
            n270 = global write "Robot Global Data.vi" "Turret Type"("Searching" ("Turret Mode")) -> ()
            n271 = global write "Robot Global Data.vi" "Auto R"(i8 0 ("Auto R")) -> ()
          }
        }
      }
      frame 8 {
        n272 = flat-sequence {
          frame #0 {
            n273 = global write "Robot Global Data.vi" "Flywheels"(TRUE ("Flywheels")) -> ()
            n274 = global write "Robot Global Data.vi" "Turret Up"(TRUE ("Flywheels")) -> ()
            n275 = global write "Robot Global Data.vi" "A Drv-R"(0.0 ("A Drv-L")) -> ()
            n276 = global write "Robot Global Data.vi" "A Drv-L"(0.0 ("A Drv-L")) -> ()
            n277 = global write "Robot Global Data.vi" "A Drv"(TRUE ("A Drv")) -> ()
            n278 = Wait (ms)(milliseconds to wait=u32 2000) -> ()  [unwired: 1 out]
          }
          frame #1 {
            n279 = global write "Robot Global Data.vi" "Fire"(TRUE ("Flywheels")) -> ()
            n280 = Wait (ms)(milliseconds to wait=u32 4000) -> ()  [unwired: 1 out]
          }
          frame #2 {
            n281 = global write "Robot Global Data.vi" "A Drv-R"(0.25 ("A Drv-L")) -> ()
            n282 = global write "Robot Global Data.vi" "A Drv-L"(-0.25 ("A Drv-L")) -> ()
            n283 = Wait (ms)(milliseconds to wait=u32 2000) -> ()  [unwired: 1 out]
          }
          frame #3 {
            n284 = global write "Robot Global Data.vi" "A Drv-R"(0.0 ("A Drv-L")) -> ()
            n285 = global write "Robot Global Data.vi" "A Drv-L"(0.0 ("A Drv-L")) -> ()
            n286 = global write "Robot Global Data.vi" "A Drv"(FALSE ("A Drv")) -> ()
            n287 = global write "Robot Global Data.vi" "Fire"(FALSE ("Flywheels")) -> ()
            n288 = global write "Robot Global Data.vi" "Auto R"(i8 0 ("Auto R")) -> ()
          }
        }
      }
      frame 9 {
        n289 = flat-sequence {
          frame #0 {
            n290 = global write "Robot Global Data.vi" "A Drv"(TRUE ("A Drv")) -> ()
            n291 = global write "Robot Global Data.vi" "Flywheels"(FALSE ("A Drv")) -> ()
            n292 = while {
              stop <- w408 stop-if-true
              n293 = global read "Robot Global Data.vi" "Drv Dist R"() -> (w407:dbl)
              n294 = global write "Robot Global Data.vi" "A Drv-R"(0.3 ("A Drv-L")) -> ()
              n295 = global write "Robot Global Data.vi" "A Drv-L"(0.3 ("A Drv-L")) -> ()
              n296 = Absolute Value(x=w407) -> (abs(x)=w406:dbl)
              n297 = Greater?(x=w406, y=1.1) -> (0:w408:bool)
            }
          }
          frame #1 {
            n298 = global write "Robot Global Data.vi" "Auto R"(i8 0 ("Auto R")) -> ()
            n299 = global write "Robot Global Data.vi" "A Drv-R"(0.0 ("A Drv-L")) -> ()
            n300 = global write "Robot Global Data.vi" "A Drv-L"(0.0 ("A Drv-L")) -> ()
            n301 = global write "Robot Global Data.vi" "A Drv"(FALSE ("A Drv")) -> ()
          }
        }
      }
    }
    n302 = Wait (ms)(milliseconds to wait=u32 100) -> ()  [unwired: 1 out]
  }
  n303 = while {
    stop <- FALSE stop-if-true
    # "Turret Adjustment and Control Functions"
    n304 = global read "Robot Global Data.vi" "Turret Type"() -> (w416:string)
    n305 = case shown="\"Semi\"" w416 {
      frame "Manual", Default {
        # "Only allows values that stay within the safe rotation range."
        n306 = global read "Robot Global Data.vi" "Turret Swiv Position"() -> (w419:dbl)
        n307 = global read "Robot Global Data.vi" "Manual Swivel Speed"() -> (w437:dbl)
        n308 = In Range and Coerce(upper limit=100, x=w419, lower limit=-100) -> (In Range?=w438:bool)  [unwired: 1 out]
        n309 = global read "Robot Global Data.vi" "Manual Swivel Speed"() -> (w434:dbl)
        n310 = global write "Robot Global Data.vi" "Tower Auto"(FALSE ("Tower Auto")) -> ()
        n311 = global read "Robot Global Data.vi" "Manual Swivel Speed"() -> (w431:dbl)
        n312 = Greater?(x=w419, y=100) -> (0:w435:bool)
        n313 = global read "Robot Global Data.vi" "Manual Swivel Speed"() -> (w426:dbl)
        n314 = Less Than 0?(x=w434) -> (x < 0?=w433:bool)
        n315 = And(x=w435, y=w433) -> (x .and. y?=w432:bool)
        n316 = global read "Robot Global Data.vi" "Manual Swivel Speed"() -> (w423:dbl)
        n317 = Less?(x=w419, y=-100) -> (x < y?=w428:bool)
        n318 = Greater Than 0?(x=w426) -> (x > 0?=w425:bool)
        n319 = And(x=w428, y=w425) -> (x .and. y?=w424:bool)
        n320 = Select(t=w423, s=w424, f=0.0) -> (s? t:f=w430:dbl)
        n321 = Select(t=w431, s=w432, f=w430) -> (s? t:f=w429:dbl)
        n322 = Select(t=w437, s=w438, f=w429) -> (s? t:f=w421:dbl)
        n323 = global write "Robot Global Data.vi" "Turret Swiv Speed"(w421) -> ()
      }
      frame "Automatic" {
        # "NOTE: Shooting Protocol still unwritten"
        n324 = global write "Robot Global Data.vi" "Tower Auto"(TRUE ("Tower Auto")) -> ()
        n325 = call-poly <vilib>:"NT Read Value.vi"("Default Value"=0.0, "Name"="/limelight/tv") -> ("Numeric"=w443:dbl)  [unwired: 8 in, 1 out]
        n326 = Equal?(x=w443, y=1.0) -> (x = y?=w442:bool)
        n327 = case shown="True" w442 {
          frame False {
            n328 = flat-sequence {
              frame #0 {
                n329 = global read "Robot Global Data.vi" "Turret Swiv Speed"() -> (w450:dbl)
                n330 = global read "Robot Global Data.vi" "Turret Swiv Speed"() -> (w447:dbl)
                n331 = Equal To 0?(x=w450) -> (x = 0?=w449:bool)
                n332 = Select(t=0.5, s=w449, f=w447) -> (s? t:f=w451:dbl)
                n333 = global write "Robot Global Data.vi" "Turret Swiv Speed"(w451) -> ()
                n334 = Wait (ms)(milliseconds to wait=u32 100) -> ()  [unwired: 1 out]
              }
              frame #1 {
                n335 = global read "Robot Global Data.vi" "Turret Swiv Position"() -> (w455:dbl)
                n336 = Absolute Value(x=w455) -> (abs(x)=w456:dbl)
                n337 = Greater?(x=w456, y=180.0) -> (0:w453:bool)
                n338 = case shown="False" w453 {
                  frame False {
                    n339 = global read "Robot Global Data.vi" "Turret Swiv Speed"() -> (w457:dbl)
                    n340 = global write "Robot Global Data.vi" "Turret Swiv Speed"(w457) -> ()
                  }
                  frame True {
                    n341 = global read "Robot Global Data.vi" "Turret Swiv Speed"() -> (w460:dbl)
                    n342 = Negate(x=w460) -> (-x=w459:dbl)
                    n343 = global write "Robot Global Data.vi" "Turret Swiv Speed"(w459) -> ()
                    n344 = Wait (ms)(milliseconds to wait=u32 1000) -> ()  [unwired: 1 out]
                  }
                }
              }
            }
          }
          frame True {
            w466 = 5.0 ("lower limit")
            w467 = -1.0 ("lower limit")
            w468 = 1.0 ("lower limit")
            w463 = -5.0 ("lower limit")
            n345 = call-poly <vilib>:"NT Read Value.vi"("Default Value"=0.0, "Name"="/limelight/tx") -> ("Numeric"=w461:dbl)  [unwired: 8 in, 1 out]
            n346 = call-poly <vilib>:"NT Read Value.vi"("Default Value"=0.0, "Name"="/limelight/tx") -> ("Numeric"=w475:dbl)  [unwired: 8 in, 1 out]
            n347 = Less?(x=w475, y=2.0) -> (x < y?=w473:bool)
            n348 = case shown="True" w473 {
              frame False {
              }
              frame True {
                n349 = global read "Robot Global Data.vi" "Target Distance"() -> (w490:dbl)
                n350 = global read "Robot Global Data.vi" "Drv Spd Av"() -> (w487:dbl)
                n351 = Less?(x=w487, y=7.0) -> (x < y?=w485:bool)
                n352 = global write "Robot Global Data.vi" "Flywheels"(w485) -> ()
                n353 = Greater?(x=w490, y=20.0) -> (0:w488:bool)
                n354 = case shown="True" w488 {
                  frame False {
                    n355 = global read "Robot Global Data.vi" "Drv Spd Av"() -> (w493:dbl)
                    n356 = Less?(x=w493, y=5.0) -> (x < y?=w491:bool)
                    n357 = global write "Robot Global Data.vi" "Fire"(w491) -> ()
                  }
                  frame True {
                    n358 = global read "Robot Global Data.vi" "Drv Spd Av"() -> (w495:dbl)
                    n359 = Equal To 0?(x=w495) -> (x = 0?=w494:bool)
                    n360 = global write "Robot Global Data.vi" "Fire"(w494) -> ()
                  }
                }
              }
            }
            n361 = In Range and Coerce(upper limit=w463, x=w461, lower limit=-20.0) -> (In Range?=w464:bool)  [unwired: 1 out]
            n362 = In Range and Coerce(upper limit=20.0 ("lower limit"), x=w461, lower limit=w466) -> (In Range?=w469:bool)  [unwired: 1 out]
            n363 = In Range and Coerce(upper limit=w466, x=w461, lower limit=w467) -> (In Range?=w471:bool)  [unwired: 1 out]
            n364 = In Range and Coerce(upper limit=w467, x=w461, lower limit=w468) -> (In Range?=w472:bool)  [unwired: 1 out]
            n365 = In Range and Coerce(upper limit=w468, x=w461, lower limit=w463) -> (In Range?=w470:bool)  [unwired: 1 out]
            n366 = case shown="True" w464 {
              frame False {
              }
              frame True {
                n367 = global write "Robot Global Data.vi" "Turret Swiv Speed"(0.3 ("Turret Swiv Speed")) -> ()
              }
            }
            n368 = case shown="True" w469 {
              frame False {
              }
              frame True {
                n369 = global write "Robot Global Data.vi" "Turret Swiv Speed"(-0.3 ("Turret Swiv Speed")) -> ()
              }
            }
            n370 = case shown="True" w471 {
              frame False {
              }
              frame True {
                n371 = global write "Robot Global Data.vi" "Turret Swiv Speed"(-0.1 ("Turret Swiv Speed")) -> ()
              }
            }
            n372 = case shown="True" w472 {
              frame False {
              }
              frame True {
                n373 = global write "Robot Global Data.vi" "Turret Swiv Speed"(0.0 ("Turret Swiv Speed")) -> ()
              }
            }
            n374 = case shown="True" w470 {
              frame False {
              }
              frame True {
                n375 = global write "Robot Global Data.vi" "Turret Swiv Speed"(0.1 ("Turret Swiv Speed")) -> ()
              }
            }
          }
        }
      }
      frame "Semi" {
        n376 = call-poly <vilib>:"NT Read Value.vi"("Default Value"=0.0, "Name"="/limelight/tv") -> ("Numeric"=w497:dbl)  [unwired: 8 in, 1 out]
        n377 = Equal?(x=w497, y=1.0) -> (x = y?=w496:bool)
        n378 = case shown="True" w496 {
          frame False {
            n379 = flat-sequence {
              frame #0 {
                n380 = global read "Robot Global Data.vi" "Turret Swiv Speed"() -> (w504:dbl)
                n381 = global read "Robot Global Data.vi" "Turret Swiv Speed"() -> (w505:dbl)
                n382 = Absolute Value(x=w504) -> (abs(x)=w503:dbl)
                n383 = Not Equal?(x=w503, y=0.5) -> (x != y?=w501:bool)
                n384 = Select(t=0.5, s=w501, f=w505) -> (s? t:f=w507:dbl)
                n385 = global write "Robot Global Data.vi" "Turret Swiv Speed"(w507) -> ()
                n386 = Wait (ms)(milliseconds to wait=u32 100) -> ()  [unwired: 1 out]
              }
              frame #1 {
                n387 = global read "Robot Global Data.vi" "Turret Swiv Position"() -> (w511:dbl)
                n388 = Absolute Value(x=w511) -> (abs(x)=w512:dbl)
                n389 = Greater?(x=w512, y=100.0) -> (0:w509:bool)
                n390 = case shown="True" w509 {
                  frame False {
                    n391 = global read "Robot Global Data.vi" "Turret Swiv Speed"() -> (w513:dbl)
                    n392 = global write "Robot Global Data.vi" "Turret Swiv Speed"(w513) -> ()
                  }
                  frame True {
                    n393 = global read "Robot Global Data.vi" "Turret Swiv Speed"() -> (w516:dbl)
                    n394 = Negate(x=w516) -> (-x=w515:dbl)
                    n395 = global write "Robot Global Data.vi" "Turret Swiv Speed"(w515) -> ()
                    n396 = Wait (ms)(milliseconds to wait=u32 1000) -> ()  [unwired: 1 out]
                  }
                }
              }
            }
          }
          frame True {
            w523 = 5.0 ("lower limit")
            w524 = -1.0 ("lower limit")
            w525 = 1.0 ("lower limit")
            w520 = -5.0 ("lower limit")
            n397 = call-poly <vilib>:"NT Read Value.vi"("Default Value"=0.0, "Name"="/limelight/tx") -> ("Numeric"=w518:dbl)  [unwired: 8 in, 1 out]
            n398 = In Range and Coerce(upper limit=w520, x=w518, lower limit=-20.0) -> (In Range?=w521:bool)  [unwired: 1 out]
            n399 = In Range and Coerce(upper limit=20.0 ("lower limit"), x=w518, lower limit=w523) -> (In Range?=w526:bool)  [unwired: 1 out]
            n400 = In Range and Coerce(upper limit=w523, x=w518, lower limit=w524) -> (In Range?=w528:bool)  [unwired: 1 out]
            n401 = In Range and Coerce(upper limit=w524, x=w518, lower limit=w525) -> (In Range?=w529:bool)  [unwired: 1 out]
            n402 = In Range and Coerce(upper limit=w525, x=w518, lower limit=w520) -> (In Range?=w527:bool)  [unwired: 1 out]
            n403 = case shown="True" w521 {
              frame False {
              }
              frame True {
                n404 = global write "Robot Global Data.vi" "Turret Swiv Speed"(0.3 ("Turret Swiv Speed")) -> ()
              }
            }
            n405 = case shown="True" w526 {
              frame False {
              }
              frame True {
                n406 = global write "Robot Global Data.vi" "Turret Swiv Speed"(-0.3 ("Turret Swiv Speed")) -> ()
              }
            }
            n407 = case shown="True" w528 {
              frame False {
              }
              frame True {
                n408 = global write "Robot Global Data.vi" "Turret Swiv Speed"(-0.1 ("Turret Swiv Speed")) -> ()
              }
            }
            n409 = case shown="True" w529 {
              frame False {
              }
              frame True {
                n410 = global write "Robot Global Data.vi" "Turret Swiv Speed"(0.0 ("Turret Swiv Speed")) -> ()
              }
            }
            n411 = case shown="True" w527 {
              frame False {
              }
              frame True {
                n412 = global write "Robot Global Data.vi" "Turret Swiv Speed"(0.1 ("Turret Swiv Speed")) -> ()
              }
            }
          }
        }
      }
    }
    n413 = Wait (ms)(milliseconds to wait=u32 100) -> ()  [unwired: 1 out]
  }
  n414 = while {
    tunnel: w20 -> [w552]
    tunnel: [w544] -> _
    tunnel: w5 -> [w547]
    tunnel: [w550] -> _
    tunnel: w3 -> [w545]
    stop <- FALSE stop-if-true
    n415 = global read "Robot Global Data.vi" "Turret Swiv Speed"() -> (w539:dbl)
    n416 = Multiply(x=w539, y=1.0) -> (x*y=w538:dbl)
    n417 = call-poly <vilib>:"CTRE_Phoenix_MotorController_Get_TalonFX.vi"("PhoenixMotorControlDevRef"=w547) -> ("Velocity (Raw Sensor Units per 100 ms)"=w548:i32)  [unwired: 11 in, 3 out]
    n418 = call-poly <vilib>:"CTRE_Phoenix_MotorController_Get_TalonFX.vi"("PhoenixMotorControlDevRef"=w545) -> ("Velocity (Raw Sensor Units per 100 ms)"=w546:i32)  [unwired: 11 in, 3 out]
    n419 = call <vilib>:"WPI_MotorControlSetOutput.vi"("Output"=w538, "MotorControlDevRef"=w552) -> ("error out"=w543:errorcluster, "MotorControlDevRef"=w544:T1)  [unwired: 7 in, 1 out]
    n420 = global read "Robot Global Data.vi" "Flywheel Speed"() -> (w551:dbl)
    n421 = global read "Robot Global Data.vi" "Flywheel Speed"() -> (w549:dbl)
    n422 = global write "Robot Global Data.vi" "Flywheel 1 Velocity"(w548) -> ()
    n423 = global write "Robot Global Data.vi" "Flywheel 2 Velocity"(w546) -> ()
    n424 = call-poly <vilib>:"CTRE_Phoenix_MotorController_Get_Enhanced.vi"("PhoenixMotorControlDevRef"=w544, "error in"=w543) -> ("Quadrature Position"=w541:i32)  [unwired: 10 in, 3 out]
    n425 = Divide(x=w541, y=122) -> (x/y=w537:dbl)
    n426 = Negate(x=w537) -> (-x=w536:dbl)
    n427 = global write "Robot Global Data.vi" "Turret Swiv Position"(w536) -> ()
    n428 = call <vilib>:"WPI_MotorControlSetOutput.vi"("Output"=w551, "MotorControlDevRef"=w547) -> ("MotorControlDevRef"=w550:T1)  [unwired: 7 in, 2 out]
    n429 = call <vilib>:"WPI_MotorControlSetOutput.vi"("Output"=w549, "MotorControlDevRef"=w545) -> ()  [unwired: 7 in, 3 out]
    n430 = Wait (ms)(milliseconds to wait=u32 100) -> ()  [unwired: 1 out]
  }
  n431 = call <vilib>:"WPI_MotorControlRefNum Registry Get.vi"("refnum name"="B_Intake") -> ("MotorControlDevRef"=w30:T1)  [unwired: 9 in, 1 out]
  n432 = while {
    stop <- FALSE stop-if-true
    n433 = global read "Robot Global Data.vi" "Intake Unjam"() -> (w555:bool)
    n434 = case shown="False" w555 {
      frame False {
        n435 = global read "Robot Global Data.vi" "Intake On"() -> (w558:bool)
        n436 = case shown="True" w558 {
          frame False {
            n437 = global write "Robot Global Data.vi" "Intake Speed"(0.0 ("Intake Speed")) -> ()
          }
          frame True {
            n438 = global write "Robot Global Data.vi" "Intake Speed"(1.0 ("Intake Speed")) -> ()
          }
        }
      }
      frame True {
        n439 = flat-sequence {
          frame #0 {
            n440 = global write "Robot Global Data.vi" "Intake Speed"(-0.6 ("Intake Speed")) -> ()
            n441 = Wait (ms)(milliseconds to wait=u32 2000) -> ()  [unwired: 1 out]
          }
          frame #1 {
            n442 = global write "Robot Global Data.vi" "Intake Speed"(0.0 ("Intake Speed")) -> ()
            n443 = global write "Robot Global Data.vi" "Intake Unjam"(FALSE ("Intake Unjam")) -> ()
          }
        }
      }
    }
    n444 = Wait (ms)(milliseconds to wait=u32 100) -> ()  [unwired: 1 out]
  }
  n445 = while {
    tunnel: w27 -> [w568]
    tunnel: [w567] -> _
    tunnel: w25 -> [w566]
    tunnel: [w565] -> _
    stop <- FALSE stop-if-true
    # "Turret firing mech. NOTE: Create turret motor speed algorithm."
    n446 = global read "Robot Global Data.vi" "Turret On"() -> (w569:bool)
    n447 = case shown="True" w569 {
      tunnel: w568 -> [w573 w578]
      tunnel: [w573 w574] -> w567
      tunnel: w566 -> [w572 w579]
      tunnel: [w572 w575] -> w565
      frame False {
      }
      frame True {
        n448 = global read "Robot Global Data.vi" "Turret Speed"() -> (w577:dbl)
        n449 = Wait (ms)(milliseconds to wait=u32 1000) -> ()  [unwired: 1 out]
        n450 = call <vilib>:"WPI_MotorControlSetOutput.vi"("Output"=w577, "MotorControlDevRef"=w579) -> ("MotorControlDevRef"=w575:T1)  [unwired: 7 in, 2 out]
        n451 = call <vilib>:"WPI_MotorControlSetOutput.vi"("Output"=w577, "MotorControlDevRef"=w578) -> ("MotorControlDevRef"=w574:T1)  [unwired: 7 in, 2 out]
      }
    }
    n452 = Wait (ms)(milliseconds to wait=u32 100) -> ()  [unwired: 1 out]
  }
  n453 = while {
    tunnel: w30 -> [w583]
    tunnel: [w582] -> _
    stop <- FALSE stop-if-true
    n454 = global read "Robot Global Data.vi" "Intake Speed"() -> (w581:dbl)
    n455 = Negate(x=w581) -> (-x=w580:dbl)
    n456 = call <vilib>:"WPI_MotorControlSetOutput.vi"("Output"=w580, "MotorControlDevRef"=w583) -> ("MotorControlDevRef"=w582:T1)  [unwired: 7 in, 2 out]
    n457 = Wait (ms)(milliseconds to wait=u32 100) -> ()  [unwired: 1 out]
  }
  n458 = disable-structure shown="Disabled" {
    frame Disabled {
      n459 = while {
        stop <- FALSE stop-if-true
        # "Center Target"
        n460 = global read "Robot Global Data.vi" "Centering TS"() -> (w586:bool)
        n461 = case shown="True" w586 {
          frame False {
          }
          frame True {
            n462 = flat-sequence {
              frame #0 {
                # "After Testing\nRemove V00 - V06"
                # "Limits Centering"
                # "Power Centering"
                n463 = global read "Robot Global Data.vi" "V00"() -> (w614:dbl)
                n464 = global read "Robot Global Data.vi" "V01"() -> (w611:dbl)
                n465 = global read "Robot Global Data.vi" "V02"() -> (w606:dbl)
                n466 = global read "Robot Global Data.vi" "V03"() -> (w603:dbl)
                n467 = global read "Robot Global Data.vi" "V04"() -> (w598:dbl)
                n468 = global read "Robot Global Data.vi" "V05"() -> (w590:dbl)
                n469 = global read "Robot Global Data.vi" "V06"() -> (w595:dbl)
                n470 = global write "Robot Global Data.vi" "A Drv"(TRUE ("Rumble")) -> ()
                n471 = global write "Robot Global Data.vi" "A Exit"(FALSE ("Rumble")) -> ()
                n472 = Add(x=0.35 ("4Bar Auto"), y=w614) -> (x+y=w615:dbl)
                n473 = Add(x=0.45 ("4Bar Auto"), y=w611) -> (x+y=w610:dbl)
                n474 = Add(x=0.6 ("4Bar Auto"), y=w606) -> (x+y=w607:dbl)
                n475 = Add(x=10.0 ("4Bar Auto"), y=w603) -> (x+y=w602:dbl)
                n476 = Add(x=90.0 ("4Bar Auto"), y=w598) -> (x+y=w599:dbl)
                n477 = Add(x=130.0 ("4Bar Auto"), y=w590) -> (x+y=w591:dbl)
                n478 = Add(x=200.0 ("4Bar Auto"), y=w595) -> (x+y=w594:dbl)
                n479 = Negate(x=w615) -> (-x=w616:dbl)
                n480 = Negate(x=w610) -> (-x=w609:dbl)
                n481 = Negate(x=w607) -> (-x=w608:dbl)
                n482 = Negate(x=w602) -> (-x=w601:dbl)
                n483 = Negate(x=w599) -> (-x=w600:dbl)
                n484 = Negate(x=w591) -> (-x=w592:dbl)
                n485 = Negate(x=w594) -> (-x=w593:dbl)
                n486 = global write "Robot Global Data.vi" "PC1"(w615) -> ()
                n487 = global write "Robot Global Data.vi" "PC2"(w616) -> ()
                n488 = global write "Robot Global Data.vi" "PC3"(w610) -> ()
                n489 = global write "Robot Global Data.vi" "PC4"(w609) -> ()
                n490 = global write "Robot Global Data.vi" "PC5"(w607) -> ()
                n491 = global write "Robot Global Data.vi" "PC6"(w608) -> ()
                n492 = global write "Robot Global Data.vi" "LC1"(w602) -> ()
                n493 = global write "Robot Global Data.vi" "LC2"(w601) -> ()
                n494 = global write "Robot Global Data.vi" "LC3"(w599) -> ()
                n495 = global write "Robot Global Data.vi" "LC4"(w600) -> ()
                n496 = global write "Robot Global Data.vi" "LC5"(w591) -> ()
                n497 = global write "Robot Global Data.vi" "LC6"(w592) -> ()
                n498 = global write "Robot Global Data.vi" "LC7"(w594) -> ()
                n499 = global write "Robot Global Data.vi" "LC8"(w593) -> ()
              }
              frame #1 {
                n500 = for {
                  N: 20 -> [_]
                  stop <- w623 stop-if-true
                  n501 = Wait (ms)(milliseconds to wait=u32 100) -> ()  [unwired: 1 out]
                  n502 = flat-sequence {
                    frame #0 {
                      n503 = for {
                        N: 20 -> [_]
                        stop <- w633 stop-if-true
                        n504 = global read "Robot Global Data.vi" "VP In View"() -> (w643:bool)
                        n505 = Wait (ms)(milliseconds to wait=u32 100) -> ()  [unwired: 1 out]
                        n506 = case shown="True" w643 {
                          frame False {
                            n507 = global write "Robot Global Data.vi" "A Drv-L"(0.0 ("4Bar Auto")) -> ()
                            n508 = global write "Robot Global Data.vi" "A Drv-R"(0.0 ("4Bar Auto")) -> ()
                          }
                          frame True {
                            n509 = global read "Robot Global Data.vi" "VP X"() -> (w655:dbl)
                            n510 = global read "Robot Global Data.vi" "LC7"() -> (w649:dbl)
                            n511 = global read "Robot Global Data.vi" "LC5"() -> (w648:dbl)
                            n512 = global read "Robot Global Data.vi" "LC3"() -> (w647:dbl)
                            n513 = global read "Robot Global Data.vi" "LC1"() -> (w654:dbl)
                            n514 = global read "Robot Global Data.vi" "LC2"() -> (w653:dbl)
                            n515 = global read "Robot Global Data.vi" "LC4"() -> (w652:dbl)
                            n516 = global read "Robot Global Data.vi" "LC6"() -> (w651:dbl)
                            n517 = global read "Robot Global Data.vi" "LC8"() -> (w650:dbl)
                            n518 = In Range and Coerce(upper limit=w649, x=w655, lower limit=w648) -> (In Range?=w660:bool)  [unwired: 1 out]
                            n519 = In Range and Coerce(upper limit=w648, x=w655, lower limit=w647) -> (In Range?=w657:bool)  [unwired: 1 out]
                            n520 = In Range and Coerce(upper limit=w647, x=w655, lower limit=w654) -> (In Range?=w661:bool)  [unwired: 1 out]
                            n521 = In Range and Coerce(upper limit=w654, x=w655, lower limit=w653) -> (In Range?=w662:bool)  [unwired: 1 out]
                            n522 = In Range and Coerce(upper limit=w653, x=w655, lower limit=w652) -> (In Range?=w659:bool)  [unwired: 1 out]
                            n523 = In Range and Coerce(upper limit=w652, x=w655, lower limit=w651) -> (In Range?=w656:bool)  [unwired: 1 out]
                            n524 = In Range and Coerce(upper limit=w651, x=w655, lower limit=w650) -> (In Range?=w658:bool)  [unwired: 1 out]
                            n525 = case shown="True" w660 {
                              frame False {
                              }
                              frame True {
                                n526 = global read "Robot Global Data.vi" "PC5"() -> (w670:dbl)
                                n527 = global write "Robot Global Data.vi" "A Drv-L"(w670) -> ()
                                n528 = global write "Robot Global Data.vi" "A Drv-R"(w670) -> ()
                              }
                            }
                            n529 = case shown="True" w657 {
                              frame False {
                              }
                              frame True {
                                n530 = global read "Robot Global Data.vi" "PC3"() -> (w664:dbl)
                                n531 = global write "Robot Global Data.vi" "A Drv-L"(w664) -> ()
                                n532 = global write "Robot Global Data.vi" "A Drv-R"(w664) -> ()
                              }
                            }
                            n533 = case shown="True" w661 {
                              frame False {
                              }
                              frame True {
                                n534 = global read "Robot Global Data.vi" "PC1"() -> (w669:dbl)
                                n535 = global write "Robot Global Data.vi" "A Drv-L"(w669) -> ()
                                n536 = global write "Robot Global Data.vi" "A Drv-R"(w669) -> ()
                              }
                            }
                            n537 = case shown="True" w662 {
                              frame False {
                              }
                              frame True {
                                w667 = 0.0 ("4Bar Auto")
                                n538 = global write "Robot Global Data.vi" "A Drv-L"(w667) -> ()
                                n539 = global write "Robot Global Data.vi" "A Drv-R"(w667) -> ()
                                n540 = global write "Robot Global Data.vi" "A Exit"(TRUE ("A Exit")) -> ()
                              }
                            }
                            n541 = case shown="True" w659 {
                              frame False {
                              }
                              frame True {
                                n542 = global read "Robot Global Data.vi" "PC2"() -> (w666:dbl)
                                n543 = global write "Robot Global Data.vi" "A Drv-L"(w666) -> ()
                                n544 = global write "Robot Global Data.vi" "A Drv-R"(w666) -> ()
                              }
                            }
                            n545 = case shown="True" w656 {
                              frame False {
                              }
                              frame True {
                                n546 = global read "Robot Global Data.vi" "PC4"() -> (w663:dbl)
                                n547 = global write "Robot Global Data.vi" "A Drv-L"(w663) -> ()
                                n548 = global write "Robot Global Data.vi" "A Drv-R"(w663) -> ()
                              }
                            }
                            n549 = case shown="True" w658 {
                              frame False {
                              }
                              frame True {
                                n550 = global read "Robot Global Data.vi" "PC6"() -> (w665:dbl)
                                n551 = global write "Robot Global Data.vi" "A Drv-L"(w665) -> ()
                                n552 = global write "Robot Global Data.vi" "A Drv-R"(w665) -> ()
                              }
                            }
                          }
                        }
                        n553 = global read "Robot Global Data.vi" "A Exit"() -> (w632:bool)
                        n554 = global read "Robot Global Data.vi" "Drv Input 1"() -> (w638:dbl)
                        n555 = global read "Robot Global Data.vi" "Drv Input 2"() -> (w636:dbl)
                        n556 = global read "Robot Global Data.vi" "Exit VP"() -> (w642:bool)
                        n557 = Absolute Value(x=w638) -> (abs(x)=w639:dbl)
                        n558 = Absolute Value(x=w636) -> (abs(x)=w637:dbl)
                        n559 = Greater?(x=w639, y=0.2) -> (0:w640:bool)
                        n560 = Greater?(x=w637, y=0.2) -> (0:w641:bool)
                        n561 = Compound Arithmetic op=OR(w632, w640, w641, w642) -> (w633:bool)
                      }
                    }
                    frame #1 {
                      n562 = global write "Robot Global Data.vi" "A Exit"(FALSE ("Rumble")) -> ()
                    }
                  }
                  n563 = global read "Robot Global Data.vi" "Drv Input 1"() -> (w627:dbl)
                  n564 = global read "Robot Global Data.vi" "Drv Input 2"() -> (w629:dbl)
                  n565 = global read "Robot Global Data.vi" "Exit VP"() -> (w620:bool)
                  n566 = Absolute Value(x=w627) -> (abs(x)=w626:dbl)
                  n567 = Absolute Value(x=w629) -> (abs(x)=w628:dbl)
                  n568 = Greater?(x=w626, y=0.2) -> (0:w622:bool)
                  n569 = Greater?(x=w628, y=0.2) -> (0:w621:bool)
                  n570 = Compound Arithmetic op=OR(w622, w621, w620) -> (w623:bool)
                }
              }
              frame #2 {
                n571 = global write "Robot Global Data.vi" "A Drv"(FALSE ("Rumble")) -> ()
                n572 = global write "Robot Global Data.vi" "A Exit"(FALSE ("Rumble")) -> ()
                n573 = global write "Robot Global Data.vi" "Centering TS"(FALSE ("Rumble")) -> ()
                n574 = global write "Robot Global Data.vi" "Precision"(TRUE ("Rumble")) -> ()
                n575 = global write "Robot Global Data.vi" "Exit VP"(FALSE ("Rumble")) -> ()
              }
            }
          }
        }
        n576 = Wait (ms)(milliseconds to wait=u32 100) -> ()  [unwired: 1 out]
      }
    }
    frame Enabled {
    }
  }
  n577 = while {
    stop <- FALSE stop-if-true
    # "Flywheels"
    n578 = global read "Robot Global Data.vi" "Required Flywheel Speed"() -> (w677:dbl)
    n579 = global read "Robot Global Data.vi" "Flywheels"() -> (w680:bool)
    n580 = Select(t=w677, s=w680, f=0.0) -> (s? t:f=w678:dbl)
    n581 = global write "Robot Global Data.vi" "Flywheel Speed"(w678) -> ()
    n582 = Wait (ms)(milliseconds to wait=u32 100) -> ()  [unwired: 1 out]
  }
  n583 = while {
    stop <- FALSE stop-if-true
    # "Turret mode handling, defaults to \"search\""
    n584 = global read "Robot Global Data.vi" "Turret Type"() -> (w683:string)
    n585 = global read "Robot Global Data.vi" "Turret Auto"() -> (w690:bool)
    n586 = global read "Robot Global Data.vi" "Turret Manual"() -> (w692:bool)
    n587 = global read "Robot Global Data.vi" "Turret Semi"() -> (w688:bool)
    n588 = Select(t="Automatic" ("Turret Mode"), s=w690, f=w683) -> (s? t:f=w684:string)
    n589 = Select(t="Semi" ("Turret Mode"), s=w688, f=w684) -> (s? t:f=w686:string)
    n590 = Select(t="Manual" ("Turret Mode"), s=w692, f=w686) -> (s? t:f=w687:string)
    n591 = global write "Robot Global Data.vi" "Turret Type"(w687) -> ()
    n592 = Wait (ms)(milliseconds to wait=u32 100) -> ()  [unwired: 1 out]
  }
  n593 = while {
    stop <- FALSE stop-if-true
    n594 = global read "Robot Global Data.vi" "Manual Roller"() -> (w697:dbl)
    n595 = Not Equal To 0?(x=w697) -> (x != 0?=w696:bool)
    n596 = case shown="False" w696 {
      frame False {
        n597 = global read "Robot Global Data.vi" "Roller Speed"() -> (w702:dbl)
        n598 = global read "Robot Global Data.vi" "Roller Speed"() -> (w708:dbl)
        n599 = Equal?(x=w702, y=-0.5) -> (x = y?=w700:bool)
        n600 = Equal?(x=w708, y=0.5) -> (x = y?=w701:bool)
        n601 = global read "Robot Global Data.vi" "Roller Speed"() -> (w704:dbl)
        n602 = Or(x=w701, y=w700) -> (x .or. y?=w699:bool)
        n603 = Select(t=0.0, s=w699, f=w704) -> (s? t:f=w706:dbl)
        n604 = global write "Robot Global Data.vi" "Roller Speed"(w706) -> ()
      }
      frame True {
        n605 = flat-sequence {
          frame #0 {
            n606 = global write "Robot Global Data.vi" "WOF Abort"(TRUE ("WOF Abort")) -> ()
          }
          frame #1 {
            n607 = global read "Robot Global Data.vi" "Manual Roller"() -> (w710:dbl)
            n608 = global write "Robot Global Data.vi" "Roller Speed"(w710) -> ()
          }
        }
      }
    }
    n609 = Wait (ms)(milliseconds to wait=u32 100) -> ()  [unwired: 1 out]
  }
  n610 = call <vilib>:"WPI_MotorControlRefNum Registry Get.vi"("refnum name"="B_Drv L1") -> ("MotorControlDevRef"=w39:T1)  [unwired: 9 in, 1 out]
  n611 = call <vilib>:"WPI_MotorControlRefNum Registry Get.vi"("refnum name"="B_Drv L2") -> ("MotorControlDevRef"=w42:T1)  [unwired: 9 in, 1 out]
  n612 = call <vilib>:"WPI_MotorControlRefNum Registry Get.vi"("refnum name"="B_Drv R1") -> ("MotorControlDevRef"=w41:T1)  [unwired: 9 in, 1 out]
  n613 = call <vilib>:"WPI_MotorControlRefNum Registry Get.vi"("refnum name"="B_Drv R2") -> ("MotorControlDevRef"=w40:T1)  [unwired: 9 in, 1 out]
  n614 = while {
    stop <- FALSE stop-if-true
    n615 = global read "Robot Global Data.vi" "Tower Auto"() -> (w711:bool)
    n616 = case shown="True" w711 {
      frame False {
      }
      frame True {
        n617 = global read "Robot Global Data.vi" "Intake On"() -> (w714:bool)
        n618 = global write "Robot Global Data.vi" "Tower Feed On"(w714) -> ()
        n619 = while {
          stop <- FALSE stop-if-true
          n620 = flat-sequence {
            frame #0 {
              n621 = global write "Robot Global Data.vi" "Shift Storage"(TRUE ("Shift Storage")) -> ()
              n622 = Wait (ms)(milliseconds to wait=u32 1000) -> ()  [unwired: 1 out]
            }
            frame #1 {
              n623 = global read "Robot Global Data.vi" "Tower LS On"() -> (w722:bool)
              n624 = while {
                stop <- w725 stop-if-true
                n625 = global read "Robot Global Data.vi" "Tower Auto"() -> (w726:bool)
                n626 = global read "Robot Global Data.vi" "Tower LS On"() -> (w723:bool)
                n627 = Not(x=w726) -> (.not. x?=w724:bool)
                n628 = Wait (ms)(milliseconds to wait=u32 100) -> ()  [unwired: 1 out]
                n629 = Or(x=w723, y=w724) -> (x .or. y?=w725:bool)
              }
              n630 = Select(t=0.0, s=w722, f=-0.5) -> (s? t:f=w719:dbl)
              n631 = global write "Robot Global Data.vi" "Tower Storage"(w719) -> ()
            }
            frame #2 {
              n632 = global write "Robot Global Data.vi" "Tower Storage"(0.0 ("Tower Storage")) -> ()
            }
          }
          n633 = Wait (ms)(milliseconds to wait=u32 100) -> ()  [unwired: 1 out]
        }
      }
    }
    n634 = Wait (ms)(milliseconds to wait=u32 100) -> ()  [unwired: 1 out]
  }
  n635 = while {
    stop <- FALSE stop-if-true
    n636 = call-poly <vilib>:"NT Read Value.vi"("Default Value"=0.0, "Name"="/limelight/ty") -> ("Numeric"=w735:dbl)  [unwired: 8 in, 1 out]
    n637 = Add(x=0.0, y=w735) -> (x+y=w730:dbl)
    n638 = expression code="(x/180.0)*pi" "degrees to radians"(w730) -> (w729:dbl)
    n639 = Subtract(x=8.1875, y=2.8958) -> (x-y=w737:dbl)
    n640 = Tangent(1:w729) -> (0:w736:dbl)
    n641 = Divide(x=w737, y=w736) -> (x/y=w734:dbl)
    n642 = Wait (ms)(milliseconds to wait=u32 100) -> ()  [unwired: 1 out]
    n643 = global write "Robot Global Data.vi" "Target Distance"(w734) -> ()
  }
  n644 = call <vilib>:"WPI_MotorControlRefNum Registry Get.vi"("refnum name"="B_ORCA Lift 1") -> ("MotorControlDevRef"=w23:T1)  [unwired: 9 in, 1 out]
  n645 = disable-structure shown="Disabled" {
    frame Disabled {
      w743 = -100.0 ("y")
      # "Accelerometer"
      # "ORCA assorted functions"
      n646 = call <vilib>:"WPI_MotorControlRefNum Registry Get.vi"("refnum name"="B_ORCA Slide") -> ("MotorControlDevRef"=w744:T1)  [unwired: 9 in, 1 out]
      n647 = call <vilib>:"WPI_AccelerometerRefNum Registry Get.vi"("refnum name"="ORCA") -> ("AccelerometerDevRef"=w742:T7)  [unwired: 9 in, 1 out]
      n648 = call <vilib>:"WPI_AccelerometerGetAcceleration.vi"("AccelerometerDevRef"=w742) -> ("Accelerations"=w747:T15)  [unwired: 8 in, 2 out]
      n649 = Unbundle By Name(w747) -> ("X-Axis"=w748:dbl, "Y-Axis"=w749:dbl, "Z-Axis"=w750:dbl)
      n650 = Multiply(x=w748, y=w743) -> (x*y=w756:dbl)
      n651 = Multiply(x=w750, y=w743) -> (x*y=w751:dbl)
      n652 = Multiply(x=w749, y=w743) -> (x*y=w755:dbl)
      n653 = Round To Nearest(number=w756) -> (nearest integer value=w752:dbl)
      n654 = Round To Nearest(number=w751) -> (nearest integer value=w754:dbl)
      n655 = Round To Nearest(number=w755) -> (nearest integer value=w753:dbl)
      n656 = global read "Robot Global Data.vi" "ORCA Wheels Man"() -> (w757:dbl)
      n657 = global write "Robot Global Data.vi" "Orca X"(w752) -> ()
      n658 = global write "Robot Global Data.vi" "Orca Y"(w753) -> ()
      n659 = global write "Robot Global Data.vi" "Orca Z"(w754) -> ()
      n660 = Greater?(x=w757, y=0.8) -> (0:w758:bool)
      n661 = case shown="True" w758 {
        tunnel: w744 -> [w762 w806]
        tunnel: [w761 w805] -> _
        frame False {
          # "Auto Pos ORCA Feedback Loop"
          n662 = global read "Robot Global Data.vi" "ORCA Align"() -> (w763:bool)
          n663 = case shown="True" w763 {
            tunnel: w762 -> [w766 w773]
            tunnel: [w766 w772] -> w761
            frame False {
              n664 = global write "Robot Global Data.vi" "ORCA Brake"(TRUE ("ORCA Brake")) -> ()
            }
            frame True {
              n665 = global read "Robot Global Data.vi" "Orca X"() -> (w788:dbl)
              n666 = global read "Robot Global Data.vi" "Orca X"() -> (w786:dbl)
              n667 = global read "Robot Global Data.vi" "Orca X"() -> (w787:dbl)
              n668 = global read "Robot Global Data.vi" "Orca X"() -> (w785:dbl)
              n669 = global read "Robot Global Data.vi" "Orca X"() -> (w784:dbl)
              n670 = In Range and Coerce(upper limit=98.0, x=w788, lower limit=95.0) -> (In Range?=w793:bool)  [unwired: 1 out]
              n671 = In Range and Coerce(upper limit=95.0, x=w787, lower limit=93.0) -> (In Range?=w790:bool)  [unwired: 1 out]
              n672 = In Range and Coerce(upper limit=93.0, x=w786, lower limit=87.0) -> (In Range?=w792:bool)  [unwired: 1 out]
              n673 = In Range and Coerce(upper limit=87.0, x=w785, lower limit=85.0) -> (In Range?=w789:bool)  [unwired: 1 out]
              n674 = In Range and Coerce(upper limit=85.0, x=w784, lower limit=80.0) -> (In Range?=w791:bool)  [unwired: 1 out]
              n675 = global read "Robot Global Data.vi" "A ORCA Wheels"() -> (w767:dbl)
              n676 = global read "Robot Global Data.vi" "Elevator Allowed"() -> (w770:bool)
              n677 = case shown="True" w793 {
                frame False {
                }
                frame True {
                  n678 = global write "Robot Global Data.vi" "A ORCA Wheels"(-0.5 ("4Bar Auto")) -> ()
                }
              }
              n679 = case shown="True" w790 {
                frame False {
                }
                frame True {
                  n680 = global write "Robot Global Data.vi" "A ORCA Wheels"(-0.25 ("4Bar Auto")) -> ()
                }
              }
              n681 = case shown="True" w792 {
                frame False {
                }
                frame True {
                  n682 = global write "Robot Global Data.vi" "A ORCA Wheels"(0.0 ("4Bar Auto")) -> ()
                  n683 = global write "Robot Global Data.vi" "ORCA Align"(FALSE ("ORCA Brake")) -> ()
                }
              }
              n684 = case shown="True" w789 {
                frame False {
                }
                frame True {
                  n685 = global write "Robot Global Data.vi" "A ORCA Wheels"(0.25 ("4Bar Auto")) -> ()
                }
              }
              n686 = case shown="True" w791 {
                frame False {
                }
                frame True {
                  n687 = global write "Robot Global Data.vi" "A ORCA Wheels"(0.5 ("4Bar Auto")) -> ()
                }
              }
              n688 = Select(t=w767, s=w770, f=0.0) -> (s? t:f=w768:dbl)
              n689 = call <vilib>:"WPI_MotorControlSetOutput.vi"("Output"=w768, "MotorControlDevRef"=w773) -> ("MotorControlDevRef"=w772:T1)  [unwired: 7 in, 2 out]
              n690 = global write "Robot Global Data.vi" "ORCA Brake"(FALSE ("ORCA Brake")) -> ()
            }
          }
          n691 = Wait (ms)(milliseconds to wait=u32 100) -> ()  [unwired: 1 out]
        }
        frame True {
          n692 = global read "Robot Global Data.vi" "ORCA Wheels Man"() -> (w801:dbl)
          n693 = global read "Robot Global Data.vi" "Elevator Allowed"() -> (w803:bool)
          n694 = Select(t=w801, s=w803, f=0.0) -> (s? t:f=w800:dbl)
          n695 = global write "Robot Global Data.vi" "ORCA Brake"(FALSE ("ORCA Brake")) -> ()
          n696 = call <vilib>:"WPI_MotorControlSetOutput.vi"("Output"=w800, "MotorControlDevRef"=w806) -> ("MotorControlDevRef"=w805:T1)  [unwired: 7 in, 2 out]
        }
      }
      n697 = Wait (ms)(milliseconds to wait=u32 100) -> ()  [unwired: 1 out]
    }
    frame Enabled {
    }
  }
  n698 = while {
    stop <- FALSE stop-if-true
    # "Wheel of Fortune Color Positioning Function"
    n699 = global read "Robot Global Data.vi" "WOF Pos"() -> (w807:bool)
    n700 = case shown="True" w807 {
      frame False {
      }
      frame True {
        n701 = global read "Robot Global Data.vi" "Challenge Color"() -> (w810:string)
        n702 = case shown="\"\", Default" w810 {
          frame "", Default {
            n703 = global write "Robot Global Data.vi" "WOF Pos"(FALSE ("WOF Pos")) -> ()
          }
          frame "Y" {
            n704 = flat-sequence {
              frame #0 {
                n705 = while {
                  stop <- w813 stop-if-true
                  n706 = global write "Robot Global Data.vi" "Roller Speed"(0.2 ("Output")) -> ()
                  n707 = global read "Robot Global Data.vi" "Color"() -> (w814:string)
                  n708 = Equal?(x=w814, y="Green" ("Color")) -> (x = y?=w813:bool)
                  n709 = Wait (ms)(milliseconds to wait=u32 10) -> ()  [unwired: 1 out]
                }
              }
              frame #1 {
                n710 = global write "Robot Global Data.vi" "WOF Pos"(FALSE ("WOF Pos")) -> ()
                n711 = global write "Robot Global Data.vi" "Roller Speed"(0.0 ("Output")) -> ()
              }
            }
          }
          frame "G" {
            n712 = flat-sequence {
              frame #0 {
                n713 = while {
                  stop <- w820 stop-if-true
                  n714 = global write "Robot Global Data.vi" "Roller Speed"(0.2 ("Output")) -> ()
                  n715 = global read "Robot Global Data.vi" "Color"() -> (w821:string)
                  n716 = Equal?(x=w821, y="Yellow" ("Color")) -> (x = y?=w820:bool)
                  n717 = Wait (ms)(milliseconds to wait=u32 10) -> ()  [unwired: 1 out]
                }
              }
              frame #1 {
                n718 = global write "Robot Global Data.vi" "WOF Pos"(FALSE ("WOF Pos")) -> ()
                n719 = global write "Robot Global Data.vi" "Roller Speed"(0.0 ("Turret Swiv Speed")) -> ()
              }
            }
          }
          frame "B" {
            n720 = flat-sequence {
              frame #0 {
                n721 = while {
                  stop <- w827 stop-if-true
                  n722 = global write "Robot Global Data.vi" "Roller Speed"(0.2 ("Output")) -> ()
                  n723 = global read "Robot Global Data.vi" "Color"() -> (w828:string)
                  n724 = Equal?(x=w828, y="Red" ("Color")) -> (x = y?=w827:bool)
                  n725 = Wait (ms)(milliseconds to wait=u32 10) -> ()  [unwired: 1 out]
                }
              }
              frame #1 {
                n726 = global write "Robot Global Data.vi" "Roller Speed"(0.0 ("Output")) -> ()
                n727 = global write "Robot Global Data.vi" "WOF Pos"(FALSE ("WOF Pos")) -> ()
              }
            }
          }
          frame "R" {
            n728 = flat-sequence {
              frame #0 {
                n729 = while {
                  stop <- w834 stop-if-true
                  n730 = global write "Robot Global Data.vi" "Roller Speed"(0.2 ("Output")) -> ()
                  n731 = global read "Robot Global Data.vi" "Color"() -> (w835:string)
                  n732 = Equal?(x=w835, y="Blue" ("Color")) -> (x = y?=w834:bool)
                  n733 = Wait (ms)(milliseconds to wait=u32 10) -> ()  [unwired: 1 out]
                }
              }
              frame #1 {
                n734 = global write "Robot Global Data.vi" "Roller Speed"(0.0 ("Output")) -> ()
                n735 = global write "Robot Global Data.vi" "WOF Pos"(FALSE ("WOF Pos")) -> ()
              }
            }
          }
        }
      }
    }
    n736 = Wait (ms)(milliseconds to wait=u32 100) -> ()  [unwired: 1 out]
  }
  n737 = while {
    stop <- FALSE stop-if-true
    # "WOF Automatic Positioning Function"
    n738 = global read "Robot Global Data.vi" "WOF Auto"() -> (w840:bool)
    n739 = case shown="True" w840 {
      frame False {
      }
      frame True {
        n740 = flat-sequence {
          frame #0 {
            n741 = global read "Robot Global Data.vi" "Color"() -> (w845:string)
            n742 = global write "Robot Global Data.vi" "Roller Speed"(0.7 ("Roller Speed")) -> ()
            n743 = global write "Robot Global Data.vi" "Auto Color Detected"(w845) -> ()
            n744 = Wait (ms)(milliseconds to wait=u32 10) -> ()  [unwired: 1 out]
          }
          frame #1 {
            n745 = while {
              stop <- w849 stop-if-true
              n746 = global read "Robot Global Data.vi" "Auto Color Detected"() -> (w851:string)
              n747 = global read "Robot Global Data.vi" "Color"() -> (w850:string)
              n748 = Equal?(x=w850, y=w851) -> (x = y?=w852:bool)
              n749 = case shown="True" w852 {
                frame False {
                }
                frame True {
                  n750 = global read "Robot Global Data.vi" "Color Counter"() -> (w856:dbl)
                  n751 = while {
                    stop <- w858 stop-if-true
                    n752 = global read "Robot Global Data.vi" "Auto Color Detected"() -> (w860:string)
                    n753 = global read "Robot Global Data.vi" "Color"() -> (w859:string)
                    n754 = Not Equal?(x=w859, y=w860) -> (x != y?=w858:bool)
                    n755 = Wait (ms)(milliseconds to wait=u32 10) -> ()  [unwired: 1 out]
                  }
                  n756 = Add(x=w856, y=1.0) -> (x+y=w854:dbl)
                  n757 = global write "Robot Global Data.vi" "Color Counter"(w854) -> ()
                  n758 = Wait (ms)(milliseconds to wait=u32 10) -> ()  [unwired: 1 out]
                }
              }
              n759 = global read "Robot Global Data.vi" "Color Counter"() -> (w848:dbl)
              n760 = Greater Or Equal?(x=w848, y=7.0) -> (x >= y?=w849:bool)
            }
            n761 = Wait (ms)(milliseconds to wait=u32 100) -> ()  [unwired: 1 out]
          }
          frame #2 {
            n762 = global write "Robot Global Data.vi" "Color Counter"(0.0 ("Color Counter")) -> ()
            n763 = global write "Robot Global Data.vi" "WOF Auto"(FALSE ("WOF Auto")) -> ()
            n764 = global write "Robot Global Data.vi" "Roller Speed"(0.0 ("Roller Speed")) -> ()
            n765 = global write "Robot Global Data.vi" "WOF Limit"(TRUE ("WOF Limit")) -> ()
            n766 = Wait (ms)(milliseconds to wait=u32 1000) -> ()  [unwired: 1 out]
          }
          frame #3 {
            n767 = global write "Robot Global Data.vi" "WOF Limit"(FALSE ("WOF Limit")) -> ()
          }
        }
      }
    }
    n768 = Wait (ms)(milliseconds to wait=u32 100) -> ()  [unwired: 1 out]
  }
  n769 = call <vilib>:"WPI_SolenoidRefNum Registry Get.vi"("refnum name"="B_Gear Shifter") -> ("SolenoidDevRef"=w22:T16)  [unwired: 9 in, 1 out]
  n770 = call <vilib>:"WPI_SolenoidRefNum Registry Get.vi"("refnum name"="B_Intake Swivel") -> ("SolenoidDevRef"=w18:T16)  [unwired: 9 in, 1 out]
  n771 = call <vilib>:"WPI_MotorControlRefNum Registry Get.vi"("refnum name"="B_Winch") -> ("MotorControlDevRef"=w1:T1)  [unwired: 9 in, 1 out]
  n772 = call <vilib>:"WPI_SolenoidRefNum Registry Get.vi"("refnum name"="B_ORCA Brake") -> ("SolenoidDevRef"=w15:T16)  [unwired: 9 in, 1 out]
  n773 = call <vilib>:"WPI_SolenoidRefNum Registry Get.vi"("refnum name"="B_Turret Vert") -> ("SolenoidDevRef"=w13:T16)  [unwired: 9 in, 1 out]
  n774 = while {
    stop <- FALSE stop-if-true
    n775 = global read "Robot Global Data.vi" "Turret Vert Value"() -> (w876:dbl)
    n776 = global read "Robot Global Data.vi" "Turret Vert Value"() -> (w873:dbl)
    n777 = global read "Robot Global Data.vi" "Turret Up"() -> (w867:bool)
    n778 = Greater?(x=w876, y=0.5) -> (0:w875:bool)
    n779 = Select(t=TRUE, s=w875, f=w867) -> (s? t:f=w870:bool)
    n780 = Less?(x=w873, y=-0.5) -> (x < y?=w871:bool)
    n781 = Select(t=FALSE, s=w871, f=w870) -> (s? t:f=w868:bool)
    n782 = global write "Robot Global Data.vi" "Turret Up"(w868) -> ()
    n783 = Wait (ms)(milliseconds to wait=u32 100) -> ()  [unwired: 1 out]
  }
  n784 = while {
    stop <- FALSE stop-if-true
    # "Turret Zero"
    n785 = global read "Robot Global Data.vi" "Brake Climb"() -> (w880:bool)
    n786 = case shown="True" w880 {
      frame False {
        n787 = global write "Robot Global Data.vi" "ORCA Brake"(FALSE ("Turret Manual")) -> ()
      }
      frame True {
        n788 = global write "Robot Global Data.vi" "ORCA Brake"(TRUE ("Turret Manual")) -> ()
      }
    }
    n789 = Wait (ms)(milliseconds to wait=u32 100) -> ()  [unwired: 1 out]
  }
  n790 = while {
    tunnel: w23 -> [w893]
    tunnel: [w892] -> _
    tunnel: w1 -> [w887]
    stop <- FALSE stop-if-true
    # "Note: Elevator Falcon 2 is inverted"
    n791 = global read "Robot Global Data.vi" "Winch Speed"() -> (w886:dbl)
    n792 = call <vilib>:"WPI_MotorControlSetOutput.vi"("Output"=w886, "MotorControlDevRef"=w887) -> ()  [unwired: 7 in, 3 out]
    n793 = global read "Robot Global Data.vi" "Winch"() -> (w885:bool)
    n794 = case shown="True" w885 {
      frame False {
        n795 = global write "Robot Global Data.vi" "Winch Speed"(0.0 ("Winch Speed")) -> ()
      }
      frame True {
        n796 = global write "Robot Global Data.vi" "Winch Speed"(-1.0 ("Winch Speed")) -> ()
      }
    }
    n797 = global read "Robot Global Data.vi" "Elevator"() -> (w888:dbl)
    n798 = Absolute Value(x=w888) -> (abs(x)=w889:dbl)
    n799 = Greater?(x=w889, y=0.5) -> (0:w890:bool)
    n800 = case shown="True" w890 {
      tunnel: w893 -> [w899 w905]
      tunnel: [w898 w901] -> w892
      frame False {
        n801 = call <vilib>:"WPI_MotorControlSetOutput.vi"("Output"=0.0, "MotorControlDevRef"=w899) -> ("MotorControlDevRef"=w898:T1)  [unwired: 7 in, 2 out]
      }
      frame True {
        n802 = global read "Robot Global Data.vi" "Elevator"() -> (w904:dbl)
        n803 = Multiply(x=w904, y=0.3) -> (x*y=w900:dbl)
        n804 = call <vilib>:"WPI_MotorControlSetOutput.vi"("Output"=w900, "MotorControlDevRef"=w905) -> ("MotorControlDevRef"=w901:T1)  [unwired: 7 in, 2 out]
        n805 = global write "Robot Global Data.vi" "Intake Down"(FALSE ("ORCA Brake")) -> ()
      }
    }
  }
  n806 = while {
    stop <- FALSE stop-if-true
    n807 = global read "Robot Global Data.vi" "Automatic Shift"() -> (w906:bool)
    n808 = case shown="False" w906 {
      frame False {
        n809 = global read "Robot Global Data.vi" "Manual High"() -> (w909:bool)
        n810 = global write "Robot Global Data.vi" "High Gear"(w909) -> ()
      }
      frame True {
      }
    }
    n811 = Wait (ms)(milliseconds to wait=u32 100) -> ()  [unwired: 1 out]
  }
  n812 = while {
    stop <- FALSE stop-if-true
    n813 = global read "Robot Global Data.vi" "Auto R"() -> (w912:i8)
    n814 = Equal?(x=w912, y=i8 0) -> (x = y?=w910:bool)
    n815 = case shown="False" w910 {
      frame False {
        n816 = global read "Robot Global Data.vi" "Turret Up"() -> (w917:bool)
        n817 = Select(t=0.37, s=w917, f=0.825) -> (s? t:f=w918:dbl)
        n818 = global write "Robot Global Data.vi" "Required Flywheel Speed"(w918) -> ()
      }
      frame True {
        n819 = global read "Robot Global Data.vi" "Turret Up"() -> (w922:bool)
        n820 = Select(t=0.37, s=w922, f=0.825) -> (s? t:f=w919:dbl)
        n821 = global write "Robot Global Data.vi" "Required Flywheel Speed"(w919) -> ()
      }
    }
    n822 = Wait (ms)(milliseconds to wait=u32 100) -> ()  [unwired: 1 out]
  }
  n823 = while {
    tunnel: w42 -> [w986]
    tunnel: w41 -> [w976]
    tunnel: w40 -> [w985]
    tunnel: [w984] -> _
    tunnel: [w983] -> _
    tunnel: [w982] -> _
    tunnel: [w981] -> _
    tunnel: w39 -> [w977]
    stop <- FALSE stop-if-true
    # "Drive System (Falcon 0, 1, 2, 3)"
    # "in Ft per Sec"
    # "Gearbox\nDirection\nCalibration"
    # "in Ft"
    # "Default averages 64 samples over 100ms"
    # "Ratios for 6\" Wheels"
    n824 = global read "Robot Global Data.vi" "Precision"() -> (w939:bool)
    n825 = global read "Robot Global Data.vi" "Automatic Shift"() -> (w940:bool)
    n826 = global read "Robot Global Data.vi" "Drive"() -> (w963:string)
    n827 = global read "Robot Global Data.vi" "D_Enc-R"() -> (w955:bool)
    n828 = Not(x=w939) -> (.not. x?=w938:bool)
    n829 = case shown="\"Cheesy\", Default" w963 {
      tunnel: [w1028 w1045 w1060] -> w972
      tunnel: [w1027 w1046 w1061] -> w971
      frame "Cheesy", Default {
        w1017 = 1.0 ("upper limit")
        w1029 = -1.0 ("lower limit")
        w1030 = -1.0 ("lower limit")
        w1031 = 1.0 ("upper limit")
        # "1 = Steering\n2 = Gas/Brake"
        # "Cheesy"
        n830 = global read "Robot Global Data.vi" "Drv Input 1"() -> (w1009:dbl)
        n831 = global read "Robot Global Data.vi" "Drv Input 2"() -> (w1010:dbl)
        n832 = global read "Robot Global Data.vi" "Drift Cal"() -> (w1011:dbl)
        n833 = global read "Robot Global Data.vi" "Turn Cal"() -> (w1008:dbl)
        n834 = Negate(x=w1010) -> (-x=w1012:dbl)
        n835 = Absolute Value(x=w1009) -> (abs(x)=w1021:dbl)
        n836 = Absolute Value(x=w1012) -> (abs(x)=w1026:dbl)
        n837 = Multiply(x=w1008, y=w1009) -> (x*y=w1018:dbl)
        n838 = Greater Or Equal?(x=w1021, y=w1011) -> (x >= y?=w1022:bool)
        n839 = Greater Or Equal?(x=w1026, y=w1011) -> (x >= y?=w1025:bool)
        n840 = Select(t=w1018, s=w1022, f=0.0) -> (s? t:f=w1019:dbl)
        n841 = Select(t=w1012, s=w1025, f=0.0) -> (s? t:f=w1020:dbl)
        n842 = In Range and Coerce(upper limit=w1031, x=w1019, lower limit=w1030) -> (coerced(x)=w1014:dbl)  [unwired: 1 out]
        n843 = In Range and Coerce(upper limit=w1031, x=w1020, lower limit=w1030) -> (coerced(x)=w1015:dbl)  [unwired: 1 out]
        n844 = Add(x=w1014, y=w1015) -> (x+y=w1016:dbl)
        n845 = Subtract(x=w1014, y=w1015) -> (x-y=w1013:dbl)
        n846 = In Range and Coerce(upper limit=w1017, x=w1016, lower limit=w1029) -> (coerced(x)=w1028:dbl)  [unwired: 1 out]
        n847 = In Range and Coerce(upper limit=w1017, x=w1013, lower limit=w1029) -> (coerced(x)=w1027:dbl)  [unwired: 1 out]
      }
      frame "Arcade" {
        w1051 = 1.0 ("upper limit")
        w1052 = -1.0 ("lower limit")
        w1053 = -1.0 ("lower limit")
        w1054 = 1.0 ("upper limit")
        # "1 = Steering\n2 = Gas/Brake"
        # "Arcade"
        n848 = global read "Robot Global Data.vi" "Drv Input 1"() -> (w1035:dbl)
        n849 = global read "Robot Global Data.vi" "Drv Input 2"() -> (w1034:dbl)
        n850 = global read "Robot Global Data.vi" "Drift Cal"() -> (w1032:dbl)
        n851 = global read "Robot Global Data.vi" "Turn Cal"() -> (w1033:dbl)
        n852 = Absolute Value(x=w1035) -> (abs(x)=w1039:dbl)
        n853 = Absolute Value(x=w1034) -> (abs(x)=w1044:dbl)
        n854 = Multiply(x=w1033, y=w1035) -> (x*y=w1038:dbl)
        n855 = Greater Or Equal?(x=w1039, y=w1032) -> (x >= y?=w1040:bool)
        n856 = Greater Or Equal?(x=w1044, y=w1032) -> (x >= y?=w1043:bool)
        n857 = Select(t=w1038, s=w1040, f=0.0) -> (s? t:f=w1036:dbl)
        n858 = Select(t=w1034, s=w1043, f=0.0) -> (s? t:f=w1037:dbl)
        n859 = In Range and Coerce(upper limit=w1054, x=w1036, lower limit=w1053) -> (coerced(x)=w1048:dbl)  [unwired: 1 out]
        n860 = In Range and Coerce(upper limit=w1054, x=w1037, lower limit=w1053) -> (coerced(x)=w1049:dbl)  [unwired: 1 out]
        n861 = Add(x=w1048, y=w1049) -> (x+y=w1050:dbl)
        n862 = Subtract(x=w1048, y=w1049) -> (x-y=w1047:dbl)
        n863 = In Range and Coerce(upper limit=w1051, x=w1050, lower limit=w1052) -> (coerced(x)=w1045:dbl)  [unwired: 1 out]
        n864 = In Range and Coerce(upper limit=w1051, x=w1047, lower limit=w1052) -> (coerced(x)=w1046:dbl)  [unwired: 1 out]
      }
      frame "Tank" {
        w1062 = 1.0 ("upper limit")
        w1063 = -1.0 ("lower limit")
        # "Tank"
        n865 = global read "Robot Global Data.vi" "Drv Input 1"() -> (w1056:dbl)
        n866 = global read "Robot Global Data.vi" "Drv Input 2"() -> (w1055:dbl)
        n867 = global read "Robot Global Data.vi" "Drift Cal"() -> (w1057:dbl)
        n868 = Absolute Value(x=w1056) -> (abs(x)=w1069:dbl)
        n869 = Absolute Value(x=w1055) -> (abs(x)=w1066:dbl)
        n870 = Greater Or Equal?(x=w1069, y=w1057) -> (x >= y?=w1068:bool)
        n871 = Greater Or Equal?(x=w1066, y=w1057) -> (x >= y?=w1067:bool)
        n872 = Select(t=w1056, s=w1068, f=0.0) -> (s? t:f=w1070:dbl)
        n873 = Select(t=w1055, s=w1067, f=0.0) -> (s? t:f=w1058:dbl)
        n874 = Negate(x=w1070) -> (-x=w1059:dbl)
        n875 = In Range and Coerce(upper limit=w1062, x=w1059, lower limit=w1063) -> (coerced(x)=w1060:dbl)  [unwired: 1 out]
        n876 = In Range and Coerce(upper limit=w1062, x=w1058, lower limit=w1063) -> (coerced(x)=w1061:dbl)  [unwired: 1 out]
      }
    }
    n877 = case shown="True" w955 {
      tunnel: w977 -> [w1072 w1079]
      tunnel: [w1072 w1078] -> w948
      tunnel: w976 -> [w1071 w1077]
      tunnel: [w1071 w1076] -> w951
      frame False {
      }
      frame True {
        n878 = global write "Robot Global Data.vi" "D_Enc-R"(FALSE ("D_Enc-R TS")) -> ()
        n879 = call-poly <vilib>:"CTRE_Phoenix_MotorControl_SetIntegratedSensorPosition_TalonFX_Polymorphic.vi"("New Position"=0.0, "PhoenixMotorControlDevRef"=w1079) -> ("PhoenixMotorControlDevRef"=w1078:T1)  [unwired: 8 in, 1 out]
        n880 = call-poly <vilib>:"CTRE_Phoenix_MotorControl_SetIntegratedSensorPosition_TalonFX_Polymorphic.vi"("New Position"=0.0, "PhoenixMotorControlDevRef"=w1077) -> ("PhoenixMotorControlDevRef"=w1076:T1)  [unwired: 8 in, 1 out]
      }
    }
    n881 = And(x=w940, y=w938) -> (x .and. y?=w937:bool)
    n882 = case shown="True" w937 {
      frame False {
      }
      frame True {
        n883 = global read "Robot Global Data.vi" "Drv Spd Av"() -> (w988:dbl)
        n884 = Absolute Value(x=w988) -> (abs(x)=w989:dbl)
        n885 = Greater Or Equal?(x=w989, y=6.0) -> (x >= y?=w990:bool)
        n886 = global write "Robot Global Data.vi" "High Gear"(w990) -> ()
      }
    }
    n887 = call-poly <vilib>:"CTRE_Phoenix_MotorController_Get_TalonFX.vi"("PhoenixMotorControlDevRef"=w948) -> ("PhoenixMotorControlDevRef"=w947:T1, "Position (Raw Sensor Units)"=w946:i32, "Velocity (Raw Sensor Units per 100 ms)"=w945:i32)  [unwired: 11 in, 1 out]
    n888 = call-poly <vilib>:"CTRE_Phoenix_MotorController_Get_TalonFX.vi"("PhoenixMotorControlDevRef"=w951) -> ("PhoenixMotorControlDevRef"=w950:T1, "Position (Raw Sensor Units)"=w926:i32, "Velocity (Raw Sensor Units per 100 ms)"=w949:i32)  [unwired: 11 in, 1 out]
    n889 = global read "Robot Global Data.vi" "High Gear"() -> (w944:bool)
    n890 = Negate(x=w946) -> (-x=w927:i32)
    n891 = global read "Robot Global Data.vi" "High Gear"() -> (w930:bool)
    n892 = Negate(x=w945) -> (-x=w974:i32)
    n893 = global read "Robot Global Data.vi" "A Drv"() -> (w954:bool)
    n894 = global read "Robot Global Data.vi" "Reverse"() -> (w962:bool)
    n895 = global read "Robot Global Data.vi" "Precision"() -> (w961:bool)
    n896 = Select(t=1037.0, s=w944, f=2133.0) -> (s? t:f=w941:dbl)
    n897 = Select(t=5000.0, s=w930, f=10500.0) -> (s? t:f=w925:dbl)
    n898 = case shown="False" w961 {
      tunnel: w972 -> [w997 w1003]
      tunnel: [w997 w1002] -> w970
      tunnel: w971 -> [w996 w1001]
      tunnel: [w996 w1000] -> w969
      frame False {
      }
      frame True {
        # "Precision\nDrive"
        n899 = Multiply(x=w1003, y=0.45 ("upper limit")) -> (x*y=w1002:dbl)
        n900 = Multiply(x=w1001, y=0.45) -> (x*y=w1000:dbl)
      }
    }
    n901 = Divide(x=w927, y=w925) -> (x/y=w923:dbl)
    n902 = Divide(x=w926, y=w925) -> (x/y=w924:dbl)
    n903 = Divide(x=w949, y=w941) -> (x/y=w957:dbl)
    n904 = Divide(x=w974, y=w941) -> (x/y=w956:dbl)
    n905 = global read "Robot Global Data.vi" "Drv-L-Out"() -> (w934:dbl)
    n906 = global read "Robot Global Data.vi" "Drv-R-Out"() -> (w933:dbl)
    n907 = Add(x=w923, y=w924) -> (x+y=w980:dbl)
    n908 = Add(x=w957, y=w956) -> (x+y=w978:dbl)
    n909 = case shown="False" w962 {
      tunnel: [w993 w995] -> w968
      tunnel: [w992 w994] -> w967
      tunnel: w970 -> [w993 w994]
      tunnel: w969 -> [w992 w995]
      frame False {
      }
      frame True {
        # "Rev"
      }
    }
    n910 = Divide(x=w980, y=2.0) -> (x/y=w959:dbl)
    n911 = Divide(x=w978, y=2.0) -> (x/y=w958:dbl)
    n912 = case shown="True" w954 {
      tunnel: [w1005 w1007] -> w966
      tunnel: [w1004 w1006] -> w965
      tunnel: w968 -> [w1005 _]
      tunnel: w967 -> [w1004 _]
      frame False {
        # "Normal\nController\nDriving"
      }
      frame True {
        # "Autonomous\nDriving"
        n913 = global read "Robot Global Data.vi" "A Drv-L"() -> (w1007:dbl)
        n914 = global read "Robot Global Data.vi" "A Drv-R"() -> (w1006:dbl)
      }
    }
    n915 = global write "Robot Global Data.vi" "Drv Dist L"(w923) -> ()
    n916 = global write "Robot Global Data.vi" "Drv Dist Av"(w959) -> ()
    n917 = global write "Robot Global Data.vi" "Drv Dist R"(w924) -> ()
    n918 = global write "Robot Global Data.vi" "Drv Spd L"(w957) -> ()
    n919 = global write "Robot Global Data.vi" "Drv Spd Av"(w958) -> ()
    n920 = global write "Robot Global Data.vi" "Drv Spd R"(w956) -> ()
    n921 = Multiply(x=w934, y=0.5) -> (x*y=w931:dbl)
    n922 = Multiply(x=w933, y=0.5) -> (x*y=w932:dbl)
    n923 = Multiply(x=w966, y=1.0) -> (x*y=w960:dbl)
    n924 = Multiply(x=w965, y=0.95) -> (x*y=w952:dbl)
    n925 = global write "Robot Global Data.vi" "Drv-L-Out"(w960) -> ()
    n926 = global write "Robot Global Data.vi" "Drv-R-Out"(w952) -> ()
    n927 = call <vilib>:"WPI_MotorControlSetOutput.vi"("Output"=w931, "MotorControlDevRef"=w947) -> ("MotorControlDevRef"=w981:T1)  [unwired: 7 in, 2 out]
    n928 = call <vilib>:"WPI_MotorControlSetOutput.vi"("Output"=w931, "MotorControlDevRef"=w986) -> ("MotorControlDevRef"=w982:T1)  [unwired: 7 in, 2 out]
    n929 = call <vilib>:"WPI_MotorControlSetOutput.vi"("Output"=w932, "MotorControlDevRef"=w950) -> ("MotorControlDevRef"=w983:T1)  [unwired: 7 in, 2 out]
    n930 = call <vilib>:"WPI_MotorControlSetOutput.vi"("Output"=w932, "MotorControlDevRef"=w985) -> ("MotorControlDevRef"=w984:T1)  [unwired: 7 in, 2 out]
    n931 = Wait (ms)(milliseconds to wait=u32 20) -> ()  [unwired: 1 out]
  }
  n932 = while {
    stop <- FALSE stop-if-true
    # "Read from Dashboard"
    n933 = call-poly <vilib>:"NT Read Value.vi"("Name"="D_W V-Array") -> ("Numeric Array"=w1108:dbl[])  [unwired: 9 in, 1 out]
    n934 = Index Array(array=w1108) -> (element #1=w1107:dbl, element #2=w1106:dbl, element #3=w1105:dbl, element #4=w1104:dbl, element #5=w1103:dbl, element #6=w1102:dbl, element #7=w1101:dbl, element #8=w1100:dbl, element #9=w1099:dbl, element #10=w1098:dbl, element #11=w1097:dbl, element #12=w1096:dbl)  [unwired: 12 in]
    n935 = global write "Robot Global Data.vi" "V00"(w1107) -> ()
    n936 = global write "Robot Global Data.vi" "V01"(w1106) -> ()
    n937 = global write "Robot Global Data.vi" "V02"(w1105) -> ()
    n938 = global write "Robot Global Data.vi" "V03"(w1104) -> ()
    n939 = global write "Robot Global Data.vi" "V04"(w1103) -> ()
    n940 = global write "Robot Global Data.vi" "V05"(w1102) -> ()
    n941 = global write "Robot Global Data.vi" "V06"(w1101) -> ()
    n942 = global write "Robot Global Data.vi" "V07"(w1100) -> ()
    n943 = global write "Robot Global Data.vi" "V08"(w1099) -> ()
    n944 = global write "Robot Global Data.vi" "V09"(w1098) -> ()
    n945 = global write "Robot Global Data.vi" "V10"(w1097) -> ()
    n946 = global write "Robot Global Data.vi" "V11"(w1096) -> ()
    n947 = call-poly <vilib>:"NT Read Value.vi"("Name"="D_W String Array") -> ("String Array"=w1094:string[])  [unwired: 9 in, 1 out]
    n948 = call-poly <vilib>:"NT Read Value.vi"("Name"="D_W Numeric Array") -> ("Numeric Array"=w1090:dbl[])  [unwired: 9 in, 1 out]
    n949 = call-poly <vilib>:"NT Read Value.vi"("Name"="D_W Boolean Array") -> ("Boolean Array"=w1083:bool[])  [unwired: 9 in, 1 out]
    n950 = Index Array(array=w1094) -> (element #1=w1093:string, element #2=w1092:string, element #3=w1091:string)  [unwired: 3 in]
    n951 = Index Array(array=w1090) -> (element #1=w1089:dbl, element #2=w1088:dbl, element #3=w1087:dbl, element #4=w1086:dbl, element #5=w1080:dbl)  [unwired: 5 in]
    n952 = Index Array(array=w1083) -> (element=w1082:bool)  [unwired: 1 in]
    n953 = global write "Robot Global Data.vi" "D_Controller"(w1093) -> ()
    n954 = global write "Robot Global Data.vi" "O_Controller"(w1092) -> ()
    n955 = global write "Robot Global Data.vi" "VP Select"(w1091) -> ()
    n956 = global write "Robot Global Data.vi" "Dash Select"(w1089) -> ()
    n957 = global write "Robot Global Data.vi" "Key Enum"(w1088) -> ()
    n958 = global write "Robot Global Data.vi" "Light Select"(w1087) -> ()
    n959 = global write "Robot Global Data.vi" "Dash X"(w1086) -> ()
    n960 = global write "Robot Global Data.vi" "CLS cal"(w1080) -> ()
    n961 = global write "Robot Global Data.vi" "Dash In View"(w1082) -> ()
    n962 = Wait (ms)(milliseconds to wait=u32 50) -> ()  [unwired: 1 out]
  }
  n963 = while {
    stop <- FALSE stop-if-true
    # "Write to Dashboard"
    n964 = global read "Robot Global Data.vi" "Turret Type"() -> (w1116:string)
    n965 = global read "Robot Global Data.vi" "Drive"() -> (w1130:string)
    n966 = Insert Into Array(array=string[] [], new element #1=w1130, new element #2=w1116) -> (w1131:string[])  [unwired: 1 in]
    n967 = call-poly <vilib>:"NT Write Value.vi"("String Array"=w1131, "Name"="D_R String Array") -> ()  [unwired: 9 in, 1 out]
    n968 = global read "Robot Global Data.vi" "Tower Feed On"() -> (w1111:bool)
    n969 = global read "Robot Global Data.vi" "Precision"() -> (w1112:bool)
    n970 = global read "Robot Global Data.vi" "High Gear"() -> (w1113:bool)
    n971 = global read "Robot Global Data.vi" "ORCA Brake"() -> (w1115:bool)
    n972 = global read "Robot Global Data.vi" "Locked On"() -> (w1118:bool)
    n973 = global read "Robot Global Data.vi" "Tower Auto"() -> (w1114:bool)
    n974 = global read "Robot Global Data.vi" "VP In View"() -> (w1117:bool)
    n975 = Insert Into Array(array=bool[] [], new element #1=w1112, new element #2=w1118, new element #3=w1117, new element #4=w1115, new element #5=w1114, new element #6=w1113, new element #7=w1111) -> (w1127:bool[])  [unwired: 1 in]
    n976 = call-poly <vilib>:"NT Write Value.vi"("Boolean Array"=w1127, "Name"="D_R Boolean Array") -> ()  [unwired: 9 in, 1 out]
    n977 = global read "Robot Global Data.vi" "Robot Lights"() -> (w1122:i8)
    n978 = global read "Robot Global Data.vi" "CamMode"() -> (w1119:i8)
    n979 = global read "Robot Global Data.vi" "VP X"() -> (w1123:dbl)
    n980 = Insert Into Array(array=dbl[] [], new element #1=w1123, new element #2=w1122, new element #3=w1119) -> (w1124:dbl[])  [unwired: 1 in]
    n981 = call-poly <vilib>:"NT Write Value.vi"("Numeric Array"=w1124, "Name"="D_R Numeric Array") -> ()  [unwired: 9 in, 1 out]
    n982 = Wait (ms)(milliseconds to wait=u32 50) -> ()  [unwired: 1 out]
  }
  n983 = while {
    tunnel: w22 -> [w1158]
    tunnel: [w1153] -> _
    tunnel: w18 -> [w1145]
    tunnel: [w1144] -> _
    tunnel: w15 -> [w1143]
    tunnel: [w1142] -> _
    tunnel: w13 -> [w1140]
    tunnel: [w1136] -> _
    stop <- FALSE stop-if-true
    n984 = global read "Robot Global Data.vi" "Turret Up"() -> (w1135:bool)
    n985 = global read "Robot Global Data.vi" "High Gear"() -> (w1157:bool)
    n986 = global read "Robot Global Data.vi" "Intake Down"() -> (w1149:bool)
    n987 = global read "Robot Global Data.vi" "ORCA Brake"() -> (w1148:bool)
    n988 = Not(x=w1135) -> (.not. x?=w1134:bool)
    n989 = Select(t=WPI_SolenoidValue."Forward" ("Value"), s=w1157, f=WPI_SolenoidValue."Reverse" ("Value")) -> (s? t:f=w1156:T18)
    n990 = Select(t=WPI_SolenoidValue."Forward" ("Value"), s=w1148, f=WPI_SolenoidValue."Reverse" ("Value")) -> (s? t:f=w1147:T18)
    n991 = Select(t=WPI_SolenoidValue."Forward" ("Value"), s=w1149, f=WPI_SolenoidValue."Reverse" ("Value")) -> (s? t:f=w1150:T18)
    n992 = Select(t=WPI_SolenoidValue."Forward" ("Value"), s=w1134, f=WPI_SolenoidValue."Reverse" ("Value")) -> (s? t:f=w1137:T18)
    n993 = call-poly <vilib>:"WPI_SolenoidSet.vi"("Value"=w1137, "SolenoidDevRef"=w1140) -> ("SolenoidDevRef"=w1136:T16)  [unwired: 8 in, 1 out]
    n994 = call-poly <vilib>:"WPI_SolenoidSet.vi"("Value"=w1156, "SolenoidDevRef"=w1158) -> ("SolenoidDevRef"=w1153:T16)  [unwired: 8 in, 1 out]
    n995 = call-poly <vilib>:"WPI_SolenoidSet.vi"("Value"=w1147, "SolenoidDevRef"=w1143) -> ("SolenoidDevRef"=w1142:T16)  [unwired: 8 in, 1 out]
    n996 = call-poly <vilib>:"WPI_SolenoidSet.vi"("Value"=w1150, "SolenoidDevRef"=w1145) -> ("SolenoidDevRef"=w1144:T16)  [unwired: 8 in, 1 out]
    n997 = Wait (ms)(milliseconds to wait=u32 100) -> ()  [unwired: 1 out]
  }
  n998 = while {
    stop <- FALSE stop-if-true
    # "Robot Light Color Change when it's Time to Climb"
    n999 = disable-structure shown="Disabled" {
      frame Disabled {
        n1000 = call <vilib>:"WPI_DriverStationGetRemainingMatchTime.vi"() -> ("Match Time(s)"=w1169:sgl)  [unwired: 10 in, 1 out]
        n1001 = global write "Robot Global Data.vi" "Match T"(w1169) -> ()
      }
      frame Enabled {
      }
    }
    n1002 = global read "Robot Global Data.vi" "Tele Time"() -> (w1161:dbl)
    n1003 = In Range and Coerce(upper limit=114.0, x=w1161, lower limit=100.0) -> (In Range?=w1164:bool)  [unwired: 1 out]
    n1004 = Greater?(x=w1161, y=115.0) -> (0:w1165:bool)
    n1005 = case shown="True" w1165 {
      frame False {
      }
      frame True {
        n1006 = global read "Robot Global Data.vi" "Light Select"() -> (w1171:i8)
        n1007 = global write "Robot Global Data.vi" "Robot Lights"(w1171) -> ()
      }
    }
    n1008 = case shown="True" w1164 {
      frame False {
      }
      frame True {
        n1009 = global write "Robot Global Data.vi" "Robot Lights"(i8 13 ("Light Select")) -> ()
      }
    }
    n1010 = Wait (ms)(milliseconds to wait=u32 100) -> ()  [unwired: 1 out]
  }
  n1011 = while {
    stop <- FALSE stop-if-true
    n1012 = global read "Robot Global Data.vi" "Man Tower Feed"() -> (w1172:bool)
    n1013 = global write "Robot Global Data.vi" "Tower Feed On"(w1172) -> ()
    n1014 = Wait (ms)(milliseconds to wait=u32 100) -> ()  [unwired: 1 out]
  }
  n1015 = call <vilib>:"WPI_MotorControlRefNum Registry Get.vi"("refnum name"="B_Storage") -> ("MotorControlDevRef"=w7:T1)  [unwired: 9 in, 1 out]
  n1016 = call <vilib>:"WPI_MotorControlRefNum Registry Get.vi"("refnum name"="B_Storage 2") -> ("MotorControlDevRef"=w8:T1)  [unwired: 9 in, 1 out]
  n1017 = call <vilib>:"WPI_MotorControlRefNum Registry Get.vi"("refnum name"="B_Shooter Feed") -> ("MotorControlDevRef"=w9:T1)  [unwired: 9 in, 1 out]
  n1018 = while {
    stop <- FALSE stop-if-true
    # "CMYK to absolute color converter"
    n1019 = global read "Robot Global Data.vi" "C Val"() -> (w1177:dbl)
    n1020 = Greater?(x=w1177, y=0.2) -> (0:w1175:bool)
    n1021 = case shown="True" w1175 {
      frame False {
        n1022 = global read "Robot Global Data.vi" "M Val"() -> (w1182:dbl)
        n1023 = Greater?(x=w1182, y=0.2) -> (0:w1180:bool)
        n1024 = case shown="True" w1180 {
          frame False {
            n1025 = global write "Robot Global Data.vi" "Color"("Undetermined" ("Color")) -> ()
          }
          frame True {
            n1026 = global write "Robot Global Data.vi" "Color"("Red" ("Color")) -> ()
          }
        }
      }
      frame True {
        n1027 = global read "Robot Global Data.vi" "C Val"() -> (w1187:dbl)
        n1028 = Greater?(x=w1187, y=0.5) -> (0:w1185:bool)
        n1029 = case shown="True" w1185 {
          frame False {
            n1030 = global write "Robot Global Data.vi" "Color"("Yellow" ("Color")) -> ()
          }
          frame True {
            n1031 = global read "Robot Global Data.vi" "Y Val"() -> (w1191:dbl)
            n1032 = Greater?(x=w1191, y=0.2) -> (0:w1189:bool)
            n1033 = case shown="True" w1189 {
              frame False {
                n1034 = global write "Robot Global Data.vi" "Color"("Blue" ("Color")) -> ()
              }
              frame True {
                n1035 = global write "Robot Global Data.vi" "Color"("Green" ("Color")) -> ()
              }
            }
          }
        }
      }
    }
    n1036 = Wait (ms)(milliseconds to wait=u32 100) -> ()  [unwired: 1 out]
  }
  n1037 = while {
    tunnel: w9 -> [w1205]
    tunnel: w8 -> [w1204]
    tunnel: w7 -> [w1203]
    tunnel: [w1198] -> _
    tunnel: [w1197] -> _
    tunnel: [w1196] -> _
    stop <- FALSE stop-if-true
    n1038 = global read "Robot Global Data.vi" "Shooter Feed"() -> (w1195:dbl)
    n1039 = global read "Robot Global Data.vi" "Tower Storage"() -> (w1202:dbl)
    n1040 = global read "Robot Global Data.vi" "Tower Feed"() -> (w1201:dbl)
    n1041 = Negate(x=w1195) -> (-x=w1194:dbl)
    n1042 = call <vilib>:"WPI_MotorControlSetOutput.vi"("Output"=w1201, "MotorControlDevRef"=w1203) -> ("MotorControlDevRef"=w1198:T1)  [unwired: 7 in, 2 out]
    n1043 = call <vilib>:"WPI_MotorControlSetOutput.vi"("Output"=w1202, "MotorControlDevRef"=w1204) -> ("MotorControlDevRef"=w1197:T1)  [unwired: 7 in, 2 out]
    n1044 = call <vilib>:"WPI_MotorControlSetOutput.vi"("Output"=w1194, "MotorControlDevRef"=w1205) -> ("MotorControlDevRef"=w1196:T1)  [unwired: 7 in, 2 out]
    n1045 = Wait (ms)(milliseconds to wait=u32 100) -> ()  [unwired: 1 out]
  }
  n1046 = while {
    stop <- FALSE stop-if-true
    n1047 = global read "Robot Global Data.vi" "Tower Feed On"() -> (w1210:bool)
    n1048 = global read "Robot Global Data.vi" "Tower Storage"() -> (w1206:dbl)
    n1049 = Select(t=1.0, s=w1210, f=w1206) -> (s? t:f=w1207:dbl)
    n1050 = Negate(x=w1207) -> (-x=w1208:dbl)
    n1051 = global write "Robot Global Data.vi" "Tower Storage"(w1207) -> ()
    n1052 = global write "Robot Global Data.vi" "Tower Feed"(w1208) -> ()
    n1053 = Wait (ms)(milliseconds to wait=u32 100) -> ()  [unwired: 1 out]
  }
  n1054 = disable-structure shown="Disabled" {
    frame Disabled {
      n1055 = call <vilib>:"WPI_PotentiometerRefNum Registry Get.vi"("refnum name"="B_Tower LS") -> ("PotDevRef"=w1214:T19)  [unwired: 9 in, 1 out]
      n1056 = while {
        tunnel: w1214 -> [w1220]
        stop <- FALSE stop-if-true
        n1057 = disable-structure shown="Disabled" {
          disable-tunnel: _ -> [w1225 _]
          disable-tunnel: [w1223 _] -> _
          disable-tunnel: [w1223 _] -> _
          frame Disabled {
            n1058 = global read "Robot Global Data.vi" "Tower LS On"() -> (w1224:bool)
            n1059 = Not Or(1:w1225, 2:w1224) -> (0:w1223:bool)
          }
          frame Enabled {
          }
        }
        n1060 = global read "Robot Global Data.vi" "Tower Auto"() -> (w1216:bool)
        n1061 = call <vilib>:"WPI_PotentiometerGetNormalized.vi"("PotDevRef"=w1220) -> ("Normalized Value"=w1219:dbl)  [unwired: 8 in, 2 out]
        n1062 = Not(x=w1216) -> (.not. x?=w1215:bool)
        n1063 = case shown="True" w1215 {
          frame False {
            n1064 = global read "Robot Global Data.vi" "Tower Auto"() -> (w1228:bool)
            n1065 = global read "Robot Global Data.vi" "Tower Feed"() -> (w1226:dbl)
            n1066 = Select(t=w1226, s=w1228) -> (s? t:f=w1227:dbl)  [unwired: 1 in]
            n1067 = global write "Robot Global Data.vi" "Tower Feed"(w1227) -> ()
          }
          frame True {
            n1068 = global read "Robot Global Data.vi" "Man Tower Feed"() -> (w1229:bool)
            n1069 = global write "Robot Global Data.vi" "Tower Feed On"(w1229) -> ()
          }
        }
        n1070 = Greater?(x=w1219, y=0.0) -> (0:w1217:bool)
        n1071 = global write "Robot Global Data.vi" "Tower LS On"(w1217) -> ()
        n1072 = Wait (ms)(milliseconds to wait=u32 100) -> ()  [unwired: 1 out]
      }
    }
    frame Enabled {
    }
  }
  n1073 = while {
    stop <- FALSE stop-if-true
    n1074 = global read "Robot Global Data.vi" "Shooter Feed On"() -> (w1230:bool)
    n1075 = case shown="True" w1230 {
      frame False {
      }
      frame True {
        n1076 = flat-sequence {
          frame #0 {
            n1077 = global write "Robot Global Data.vi" "Shooter Feed"(1.0 ("Shooter Feed")) -> ()
            n1078 = Wait (ms)(milliseconds to wait=u32 2000) -> ()  [unwired: 1 out]
          }
          frame #1 {
            n1079 = global write "Robot Global Data.vi" "Shooter Feed On"(FALSE ("Shooter Feed On")) -> ()
            n1080 = global write "Robot Global Data.vi" "Shooter Feed"(0.0 ("Shooter Feed")) -> ()
          }
        }
      }
    }
    n1081 = Wait (ms)(milliseconds to wait=u32 100) -> ()  [unwired: 1 out]
  }
  n1082 = call <vilib>:"WPI_MotorControlRefNum Registry Get.vi"("refnum name"="B_Lights") -> ("MotorControlDevRef"=w33:T1)  [unwired: 9 in, 1 out]
  n1083 = while {
    stop <- FALSE stop-if-true
    n1084 = global read "Robot Global Data.vi" "Tower Unjam"() -> (w1237:bool)
    n1085 = case shown="True" w1237 {
      frame False {
      }
      frame True {
        n1086 = flat-sequence {
          frame #0 {
            w1241 = -1.0 ("Tower Storage")
            n1087 = global write "Robot Global Data.vi" "Tower Storage"(w1241) -> ()
            n1088 = global write "Robot Global Data.vi" "Shooter Feed"(w1241) -> ()
            n1089 = global write "Robot Global Data.vi" "Tower Feed"(w1241) -> ()
            n1090 = Wait (ms)(milliseconds to wait=u32 1500) -> ()  [unwired: 1 out]
          }
          frame #1 {
            w1242 = 0.0 ("Tower Storage")
            n1091 = global write "Robot Global Data.vi" "Tower Unjam"(FALSE ("Tower Unjam")) -> ()
            n1092 = global write "Robot Global Data.vi" "Tower Storage"(w1242) -> ()
            n1093 = global write "Robot Global Data.vi" "Shooter Feed"(w1242) -> ()
            n1094 = global write "Robot Global Data.vi" "Tower Feed"(w1242) -> ()
          }
        }
      }
    }
    n1095 = Wait (ms)(milliseconds to wait=u32 100) -> ()  [unwired: 1 out]
  }
  n1096 = while {
    tunnel: w33 -> [w1245]
    tunnel: [w1244] -> _
    stop <- FALSE stop-if-true
    # "Robot Lights (PWM 9)"
    n1097 = global read "Robot Global Data.vi" "Robot Lights"() -> (w1248:i8)
    n1098 = Multiply(x=w1248, y=0.0625 ("PWM Divide")) -> (x*y=w1247:dbl)
    n1099 = Subtract(x=w1247, y=1.0) -> (x-y=w1249:dbl)
    n1100 = call <vilib>:"WPI_MotorControlSetOutput.vi"("Output"=w1249, "MotorControlDevRef"=w1245) -> ("MotorControlDevRef"=w1244:T1)  [unwired: 7 in, 2 out]
    n1101 = Wait (ms)(milliseconds to wait=u32 100) -> ()  [unwired: 1 out]
  }
  n1102 = disable-structure shown="Disabled" {
    frame Disabled {
      n1103 = while {
        stop <- FALSE stop-if-true
        n1104 = global read "Robot Global Data.vi" "Tower Feed On"() -> (w1254:bool)
        n1105 = global read "Robot Global Data.vi" "Tower LS On"() -> (w1256:bool)
        n1106 = Not(x=w1256) -> (.not. x?=w1255:bool)
        n1107 = And(x=w1255, y=w1254) -> (x .and. y?=w1253:bool)
        n1108 = case shown="True" w1253 {
          frame False {
          }
          frame True {
            n1109 = flat-sequence {
              frame #0 {
                n1110 = Wait (ms)(milliseconds to wait=u32 3000) -> ()  [unwired: 1 out]
              }
              frame #1 {
                n1111 = global read "Robot Global Data.vi" "Tower LS On"() -> (w1261:bool)
                n1112 = Wait (ms)(milliseconds to wait=u32 100) -> ()  [unwired: 1 out]
                n1113 = case shown="True" w1261 {
                  frame False {
                  }
                  frame True {
                    n1114 = global write "Robot Global Data.vi" "Ball Taken"(TRUE ("Ball Taken")) -> ()
                  }
                }
              }
              frame #2 {
                n1115 = global write "Robot Global Data.vi" "Ball Taken"(FALSE ("Ball Taken")) -> ()
              }
            }
          }
        }
        n1116 = Wait (ms)(milliseconds to wait=u32 100) -> ()  [unwired: 1 out]
      }
      n1117 = while {
        stop <- FALSE stop-if-true
        # "Cell Counter"
        n1118 = global read "Robot Global Data.vi" "Flywheels"() -> (w1266:bool)
        n1119 = global read "Robot Global Data.vi" "Fire"() -> (w1265:bool)
        n1120 = global read "Robot Global Data.vi" "Cell Counter"() -> (w1270:dbl)
        n1121 = global read "Robot Global Data.vi" "Ball Taken"() -> (w1267:bool)
        n1122 = global read "Robot Global Data.vi" "Cell Counter"() -> (w1275:dbl)
        n1123 = global read "Robot Global Data.vi" "Cell Counter"() -> (w1268:dbl)
        n1124 = And(x=w1265, y=w1266) -> (x .and. y?=w1264:bool)
        n1125 = Add(x=w1270, y=1.0) -> (x+y=w1269:dbl)
        n1126 = Subtract(x=w1275, y=1.0) -> (x-y=w1273:dbl)
        n1127 = Select(t=w1269, s=w1267, f=w1268) -> (s? t:f=w1272:dbl)
        n1128 = Select(t=w1273, s=w1264, f=w1272) -> (s? t:f=w1276:dbl)
        n1129 = global write "Robot Global Data.vi" "Cell Counter"(w1276) -> ()
        n1130 = Wait (ms)(milliseconds to wait=u32 100) -> ()  [unwired: 1 out]
      }
    }
    frame Enabled {
    }
  }
  n1131 = call <vilib>:"WPI_JoystickRefNum Registry Get.vi"("refnum name"="B_Driver") -> ("JoystickDevRef"=w31:T20)  [unwired: 9 in, 1 out]
  n1132 = while {
    stop <- FALSE stop-if-true
    n1133 = call <vilib>:"WPI_DriverStationGame Specific Data.vi"() -> ("Game Specific Data"=w1279:string)  [unwired: 11 in]
    n1134 = global write "Robot Global Data.vi" "Challenge Color"(w1279) -> ()
    n1135 = Wait (ms)(milliseconds to wait=u32 100) -> ()  [unwired: 1 out]
  }
  n1136 = disable-structure shown="Disabled" {
    frame Disabled {
      n1137 = call <vilib>:"Color Sensor V3 RefNum Registry Get.vi"("refnum name"="ColorSensor") -> ("ColorSensorDevRef"=w1282:T22)  [unwired: 9 in, 1 out]
      n1138 = while {
        tunnel: w1282 -> [w1293]
        stop <- FALSE stop-if-true
        n1139 = call <vilib>:"Color Sensor V3 Get Color.vi"("ColorSensorDevRef"=w1293) -> ("Color"=w1292:u32)  [unwired: 7 in, 3 out]
        n1140 = call <vilib>:"Color to RGB.vi"("Color"=w1292) -> ("R"=w1291:u8, "G"=w1290:u8, "B"=w1289:u8)  [unwired: 1 out]
        n1141 = formula code="C = 1 - ( R / 255 );\nM = 1 - ( G / 255 );\nY = 1 - ( B / 255 );\nK=1;\n\nif ( C < K )   K = C;\nif ( M < K )   K = M;\nif ( Y < K )   K = Y;\n\nif ( K == 1 ) //Black\n{ C = 0;\n   M = 0;\n   Y = 0;}\n\nelse\n{  C = ( C - K ) / ( 1 - K );\n    M = ( M - K ) / ( 1 - K );\n    Y = ( Y - K ) / ( 1 - K );}"("R"=w1291, "G"=w1290, "B"=w1289) -> ("C"=w1287:dbl, "M"=w1286:dbl, "Y"=w1285:dbl)  [unwired: 1 out]
        n1142 = global write "Robot Global Data.vi" "Y Val"(w1285) -> ()
        n1143 = global write "Robot Global Data.vi" "M Val"(w1286) -> ()
        n1144 = global write "Robot Global Data.vi" "C Val"(w1287) -> ()
        n1145 = Wait (ms)(milliseconds to wait=u32 100) -> ()  [unwired: 1 out]
      }
    }
    frame Enabled {
    }
  }
  n1146 = while {
    stop <- FALSE stop-if-true
    # "Rumble at 30 Secs Left in Match"
    n1147 = global read "Robot Global Data.vi" "Tele Time"() -> (w1297:dbl)
    n1148 = In Range and Coerce(upper limit=90.5, x=w1297, lower limit=90.0) -> (In Range?=w1294:bool)  [unwired: 1 out]
    n1149 = case shown="True" w1294 {
      frame False {
      }
      frame True {
        n1150 = flat-sequence {
          frame #0 {
            n1151 = global write "Robot Global Data.vi" "Rumble"(TRUE ("Rumble")) -> ()
            n1152 = Wait (ms)(milliseconds to wait=u32 1000) -> ()  [unwired: 1 out]
          }
          frame #1 {
            n1153 = global write "Robot Global Data.vi" "Rumble"(FALSE ("Rumble")) -> ()
          }
        }
      }
    }
    n1154 = Wait (ms)(milliseconds to wait=u32 200) -> ()  [unwired: 1 out]
  }
  n1155 = while {
    tunnel: w31 -> [w1303]
    stop <- FALSE stop-if-true
    # "Rumble Driver Controller"
    n1156 = global read "Robot Global Data.vi" "Rumble"() -> (w1304:bool)
    n1157 = case shown="True" w1304 {
      tunnel: w1303 -> [w1307 w1310]
      frame False {
        w1308 = sgl 0.0 ("Left Rumble")
        n1158 = call <vilib>:"WPI_JoystickSetOutputs.vi"("Right Rumble"=w1308, "Left Rumble"=w1308, "JoystickDevRef"=w1307) -> ()  [unwired: 7 in, 2 out]
      }
      frame True {
        w1309 = sgl 1.0 ("Left Rumble")
        n1159 = call <vilib>:"WPI_JoystickSetOutputs.vi"("Right Rumble"=w1309, "Left Rumble"=w1309, "JoystickDevRef"=w1310) -> ()  [unwired: 7 in, 2 out]
      }
    }
    n1160 = Wait (ms)(milliseconds to wait=u32 100) -> ()  [unwired: 1 out]
  }
  n1161 = disable-structure shown="Disabled" {
    frame Disabled {
      (unwired) "This VI is a good place to take care of periodic tasks such as control loops.\n\nAdd code to the existing loops, or duplicate a loop to define a new rate. You can allocate I/O references here, or in Begin.vi.\n\nPeriodic loops will often operate with setpoints from other loops. Use a global variable such as Robot Global Data for sharing data between loops."
      n1162 = call <vilib>:"WPI_JoystickRefNum Registry Get.vi"("refnum name"="Joystick 0") -> ("JoystickDevRef"=w1313:T20)  [unwired: 1 in, 9 out]
      n1163 = call <vilib>:"WPI_RobotDriveRefNum Registry Get.vi"("refnum name"="Left and Right Motors") -> ("RobotDriveDevRef"=w1312:T24)  [unwired: 1 in, 9 out]
      n1164 = Bundle("JoystickDevRef"=w1313, "RobotDriveDevRef"=w1312) -> (w1311:T25)  [unwired: 1 out]
      n1165 = while {
        shift-right: [w1319] -> _
        shift-left: w1311 -> [w1319]
        stop <- FALSE stop-if-true
        # "10 ms tasks go here"
        n1166 = Wait (ms)(milliseconds to wait=u32 10) -> ()  [unwired: 1 out]
      }
      n1167 = while {
        shift-right: [w1316] -> _
        shift-left: w1311 -> [w1316]
        stop <- FALSE stop-if-true
        # "100 ms tasks go here"
        n1168 = Wait (ms)(milliseconds to wait=u32 100) -> ()  [unwired: 1 out]
      }
    }
    frame Enabled {
    }
  }
